vi "Software Echarpe.vi"() -> ()   [LabVIEW 2012]
doc: "Este é o VI principal que contém a interface de controle do espectrógrafo e demais intrumentos."
uses:
  Application/Application.lvclass
  Application/Application.lvclass/Application.ctl
  RxTx/RxTx.lvclass/RxTx.ctl
  Setup File/Setup File.lvclass/Setup File.ctl
  Display Image/Display Image.lvclass/Display Image.ctl
  CCDCamera/CCDCamera.lvclass/CCDCamera.ctl
  Instrument/Instrument.lvclass/Instrument.ctl
  Setup File/Setup File.lvclass
  Display Image/Display Image.lvclass
  CCDCamera/CCDCamera.lvclass
  RxTXCamera/RxTxCamera.lvclass
  State Machine/State Machine.lvclass
  User/User.lvclass
  TCS/TCS.lvclass
  Guider/Guider.lvclass
  Calibration Unit/Calibration Unit.lvclass
  Weather Station/Weather Station.lvclass
  Fore Optics/Fore Optics.lvclass
  Dome/Dome.lvclass
  Instrument/Instrument.lvclass
  RxTx/RxTx.lvclass
panel:
  in  "Image Format":string
  in  "Clean Error":bool
  in  "Application.lvclass":refnum<class "Application.lvclass">
  in  "Night Directory":string="C:\\Users\\Sparc4_2\\Desktop\\Software Echarpe\\Imagens"
  in  "Program ID":string="UNDEFINED"
  in  "Object":string="UNDEFINED"
  in  "Observer":string="ECHARPE"
  in  "Texp Azul":dbl
  in  "Texp Vermelho":dbl
  in  "Posição do rotor":dbl
  in  "Ângulo de paralaxe":dbl
  in  "Blank Button 7":bool
  in  "Blank Button 6":bool
  out "Guiando":bool=TRUE
  out "Waveform Graph":dbl[](graph)
  out "Intensity Graph 4":dbl[][](graph)
  out "Date":string="04/05/2018"
  out "UT":string="2017-10-01T20:34:3 6.000"
  out "Sidereal Time":string="2017-10-01T20:34:3 6.000"
  out "Focus":string="-3.53"
  out "PA":string="14.6415392418"
  out "HA":string="+01:13:05.98"
  out "DEC":string="+00:00:00.000"
  out "Air Mass":string="1.085"
  out "RA":string="00:00:00.000"
  in  "Stop Button":bool
  in  "Interface de controle":T1(tab)
  in  "Pausar":bool
  out "Temperature":i16
  out "Initialization":bool
  out "% Acquired":dbl
  out "Exposing":bool=TRUE
  out "Exposições realizadas":u8(slide) scale=0.0..100.0
  in  "Image Name":string
  in  "# Exposure":dbl
  in  "Exposure time":dbl
  out "% Acquired":dbl
  out "LED sky":bool
  in  "Sky Fiber":bool
  out "LED cal":bool
  in  "Calibration Fiber":bool
  out "Setup File Path:":string
  in  "Read mode":enum32{"No Selection", "1", "2", "3"}(radio)=enum."1"
  in  "Load Setup":bool
  in  "COMP":bool
  in  "FLAT":bool
  in  "Sync Mode":bool
  in  "Adquirir 4":bool
  out "Exposing":bool
  out "Exposições realizadas":u8(slide) scale=0.0..1.0
  in  "Data:":dbl
  in  "Y :":dbl
  in  "X :":dbl
  out "Data:":u32
  out "Y :":u16
  in  "Pausar 3":bool
  in  "Stop 3":bool
  in  "Abort 3":bool
  in  "Adquirir 3":bool
  in  "Pausar 2":bool
  in  "Stop 2":bool
  in  "Stop":bool
  in  "Abort 2":bool
  in  "Adquirir":bool
  in  "Abort":bool
  out "Last Image":string
  in  "# Exposure":u32=1 min=1
  in  "Exposure time":dbl min=0.0
  out "Intensity Graph 2":dbl[][](graph)
  in  "BIAS":bool
  out "X :":u16
  out "Error led":bool
  out "Error Num":u16
  out "Error string":string
  out "Error led 2":bool
  out "Error string 2":string
  out "Error Num 2":u16
  out "Image Graph":i32[][](graph)
  in  "Load Seup 2":bool
  in  "Save Setup":bool
  in  "Tab Control":T2(tab)
  in  "RED Channel Setup":enum32{"Setup", "Binning", "Saving "}(tab)
  in  "Exposure Time (s)  2":dbl
  in  "Acquisition Mode":u16(ring)=1 items=["RESERVED", "Single Scan", "Accumulate", "Kinetics", "Fast Kinetics", "Run Til Abort", "RESERVED", "RESERVED", "RESERVED", "RESERVED", "Time Delayed Integration"]
  in  "Read Mode":u16(ring)=4 items=["Full Vertical Binning", "Multi-Track", "Random-Track", "Single-Track", "Image"]
  in  "Trigger":u16(ring) items=["Internal", "External", "N/A", "N/A", "N/A", "N/A", "External Start", "External Exposure (bulb)", "N/A", "External FVB EM", "Software", "N/A", "External Charge Shifting"]
  in  "Readout Rate":u8(ring) items=["100 KHz at 16 bit", "1 MHz at 16 bit"]
  in  "Vertical Shift Speed":u8(ring) items=["0.6", "2.2", "3.6", "4.33"]
  in  "Vertical clock\nvoltage amplitude":u8
  in  "Pre-amplifier gain":u8(ring)=1 items=["1", "2", "4"]
  in  "Time to close (ms)":u16=50 min=50
  in  "Time to open (ms)":u16=50 min=50
  in  "Shutter TTL":u16(ring) items=["TTL Low", "TTL High"]
  in  "Shutter Mode":u16(ring)=2 items=["Fully Auto", "OPEN", "CLOSED"]
  out "Temperature ºC":dbl(slide) min=-120.0 max=20.0
  in  "Set temperature":i8=20 min=0 max=0
  in  "Cooler ON/OFF":u16(ring) items=["Cooler OFF", "Cooler ON"]
  in  "Vertical binning":u16=1 min=1
  in  "Horizontal binning":u16=1 min=1
  in  "Final Column":u16=1024 min=1
  in  "Final Line":u16=1024 min=1
  in  "Initial Column":u16=1 min=1
  in  "Initial Line":u16=1 min=1
  in  "Sub Image":T3(radio)=enum."1024 x 1024"
  out "Binning":cluster{dbl, dbl}[](graph)
  in  "FITS Format":u16(ring) items=["Unsigned 16", "Unsigned 32", "Signed 16", "Signed 32", "Float"]
  in  "FITS":bool
  in  "SIF":bool
  in  "TIFF":bool
  in  "Tiff Type":u16(ring) items=["8-bit", "16-bit", "Color"]
  in  "Tiff Position":u16=1
  in  "Exposure Time (s)":sgl format="%.2f"
  in  "Acquisition Mode":u16(ring)=1 items=["RESERVED", "Single Scan", "Accumulate", "Kinetics", "Fast Kinetics", "Run Til Abort", "RESERVED", "RESERVED", "RESERVED", "RESERVED", "Time Delayed Integration"]
  in  "Read Mode":u16(ring)=4 items=["Full Vertical Binning", "Multi-Track", "Random-Track", "Single-Track", "Image"]
  in  "Conventional/EM":i32(ring) items=["Conventional", "EM Gain"]
  in  "Trigger":u16(ring) items=["Internal", "External", "N/A", "N/A", "N/A", "N/A", "External Start", "External Exposure (bulb)", "N/A", "External FVB EM", "Software", "N/A", "External Charge Shifting"]
  in  "Readout Rate":i32
  in  "Vertical Shift Speed":i32
  in  "Vertical clock\n  voltage amplitude":i32
  in  "Pre-amplifier gain":i32=1
  in  "EM Gain":bool
  in  "EM Gain  level":i32=1
  in  "EM Advanced 3":bool
  in  "Baseline Clamp 3":bool
  in  "Time to close (ms)":dbl=50.0
  in  "Time to open (ms)":dbl=50.0
  in  "Shutter TTL":u16(ring) items=["TTL Low", "TTL High"]
  in  "Shutter Mode":u16(ring)=2 items=["Fully Auto", "OPEN", "CLOSED"]
  out "Temperature ºC":dbl(slide) scale=-100.0..30.0
  in  "Set temperature":dbl=20.0 min=-80.0 max=20.0
  in  "Cooler ON/OFF":u16(ring) items=["Cooler OFF", "Cooler ON"]
  # "Error Message"
  # "Error Message"
  # "Sync Mode"
  # "Bias"
  # "Flat"
  # "Comp"
  # "RED Channel"
  # "Set Shutter Configuration"
  # "Timings"
  # "Vertical pixel shift"
  # "(TTL level required \nto open  your \nexternal shutter)"
  # "Time to open/close shutter"
  # "Horizontal pixel shift"
  # "Temperature"
  # "Save As:"
  # "BLUE Channel"
  # "Set Shutter Configuration"
  # "Timings"
  # "Vertical pixel shift"
  # "(TTL level required to open \nyour external shutter)"
  # "Time to open/close shutter"
  # "Horizontal pixel shift"
  # "Temperature"
  # "Electron Multiplier (EM) Gain"
  # "Baseline"
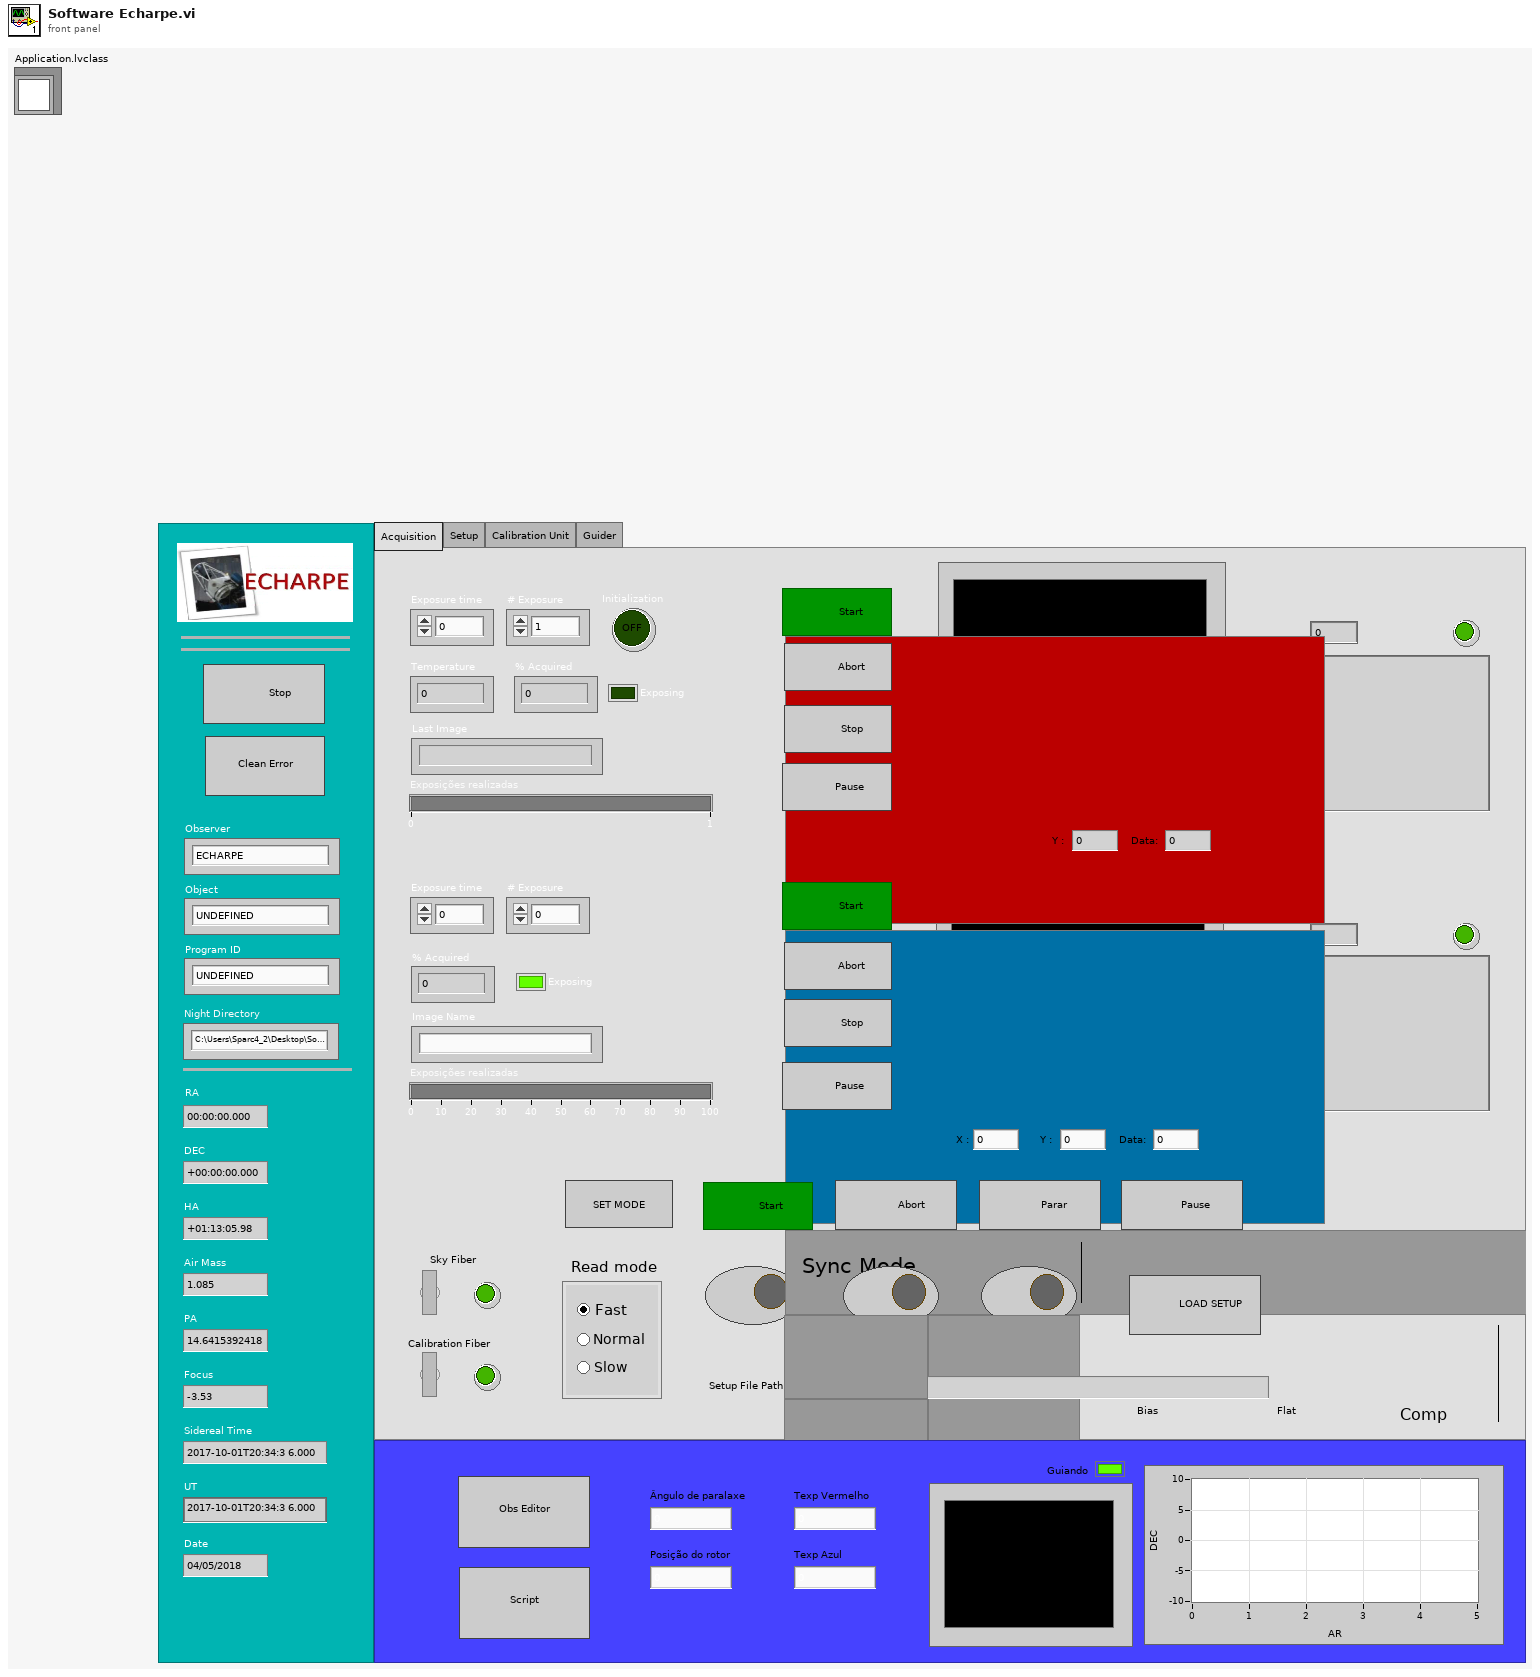
[diagram p1: front panel]
types:
  T1 = enum32{"Acquisition", "Setup", "Calibration Unit", "Guider"}
  T2 = enum32{"RED Channel", "BLUE Channel", "Instrument"}
  T3 = enum32{"256 x 256", "512 x 512", "1024 x 1024", "Custom", "128 x 128", "64 x 64"}
  T4 = cluster{"Currently Temperature":dbl, "Last Image":string, "% Acquired":dbl, "Initilizarion":bool, "Exposing":bool, "Temperature Status":string, "X length":dbl, "Y length":dbl, "Min Temperature":dbl, "Max Temperature":dbl}
  T5 = cluster{"BIAS":refnum<vi>, "FLAT":refnum<vi>, "COMP":refnum<vi>, "Read mode":refnum<vi>}
  T6 = cluster{"Shutter Mode ":u16, "Pre-amplifier gain":i32, "Vertical Shift Speed":i32, "Readout Rate ":i32, "Exposure Time (s) ":sgl}
  T7 = cluster{"Cooler ON/OFF":u16, "Set temperature":dbl, "Shutter Mode ":u16, "Shutter TTL":u16, "Time to open (ms)":dbl, "Time to close (ms)":dbl, "Pre-amplifier gain":i32, "Vertical clock\n  voltage amplitude":i32, "Vertical Shift Speed":i32, "Readout Rate ":i32, "Trigger ":u16, "Conventional/EM":i32, "Read Mode ":u16, "Acquisition Mode ":u16, "Exposure Time (s) ":sgl, "Initial Line":i32, "Initial Column":i32, "Final Line":i32, "Final Column":i32, "Horizontal binning":i32, "Vertical binning ":i32, "FITS Format":u16, "Image Format":string, "Tiff Position ":u16, "Tiff Type":u16, "Image Path":string}
  T8 = cluster{"DSTATUS":string, "DPOS":string, "DTEMP":string, "DHUM":string, "DLAMP":string, "DFLAT":string}
  T9 = cluster{"ADC":string, "ADCSPEED":string, "CALMIRR":string}
  T10 = cluster{"TEMPEXT":string, "PRESSURE":string, "HUMIDITY":string, "WINDDIR":string, "WSPEED":string}
  T11 = cluster{"THARLAMP":string, "HALLAMP":string, "AGITATOR":string, "THARMIRR":string}
  T12 = cluster{"GUIDING":string, "GUIDTEXP":string, "GUIDFREQ":string, "GUIDOBJX":string, "GUIDOBJY":string, "AVGYCOOR":string, "AVGXCORR":string, "GFOCUS":string}
  T13 = cluster{"Observation type":string, "Read Mode":string, "Sky fiber":bool, "Calibration fiber":bool, "Sync Mode":string, "Date":string}
  T14 = cluster{"RA":string, "DEC":string, "TELRA":string, "TELDEC":string, "RA_DEG":string, "DEC_DEG":string, "Epoch":string, "AirMass":string, "Initial Air Mass":string, "HA":string, "HAD":string, "Final Air Mass":string, "X Offset":string, "Y Offset":string, "PA":string, "Camera Focus":string, "TCS Focus":string, "Moon distance":string, "Moon height":string, "Moon Phase":string, "TCSST":string, "TCSUT":string}
  T15 = cluster{"Observer":string, "Object":string, "Program ID":string, "Night Directory":string}
  T16 = cluster{"Read Mode":string, "Acquisition Mode":string, "Trigger":string, "Exposure Time":string, "VShift Speed":string, "Readout rate":string, "Pre amp":string, "Shutter Mode":string, "Shutter TTL":string, "Time to open shutter":string, "Time to close shutter":string, "Cooler":string, "Temperature":string, "Initial Line":string, "Initial Column":string, "Final Line":string, "Final Column":string, "Horizontal binning":string, "Vertical binning":string, "Sub image":string}
  T17 = enum8{"Enabled", "Disabled", "Disabled and Grayed Out"}
  T18 = cluster{"Exposing":bool, "% Acquired":dbl, "Initialization":bool, "CurrentlyTemp":i16, "Exposições realizadas":u8, "Image Graph":i32[][], "Temperature Status":string, "Last Image":string}
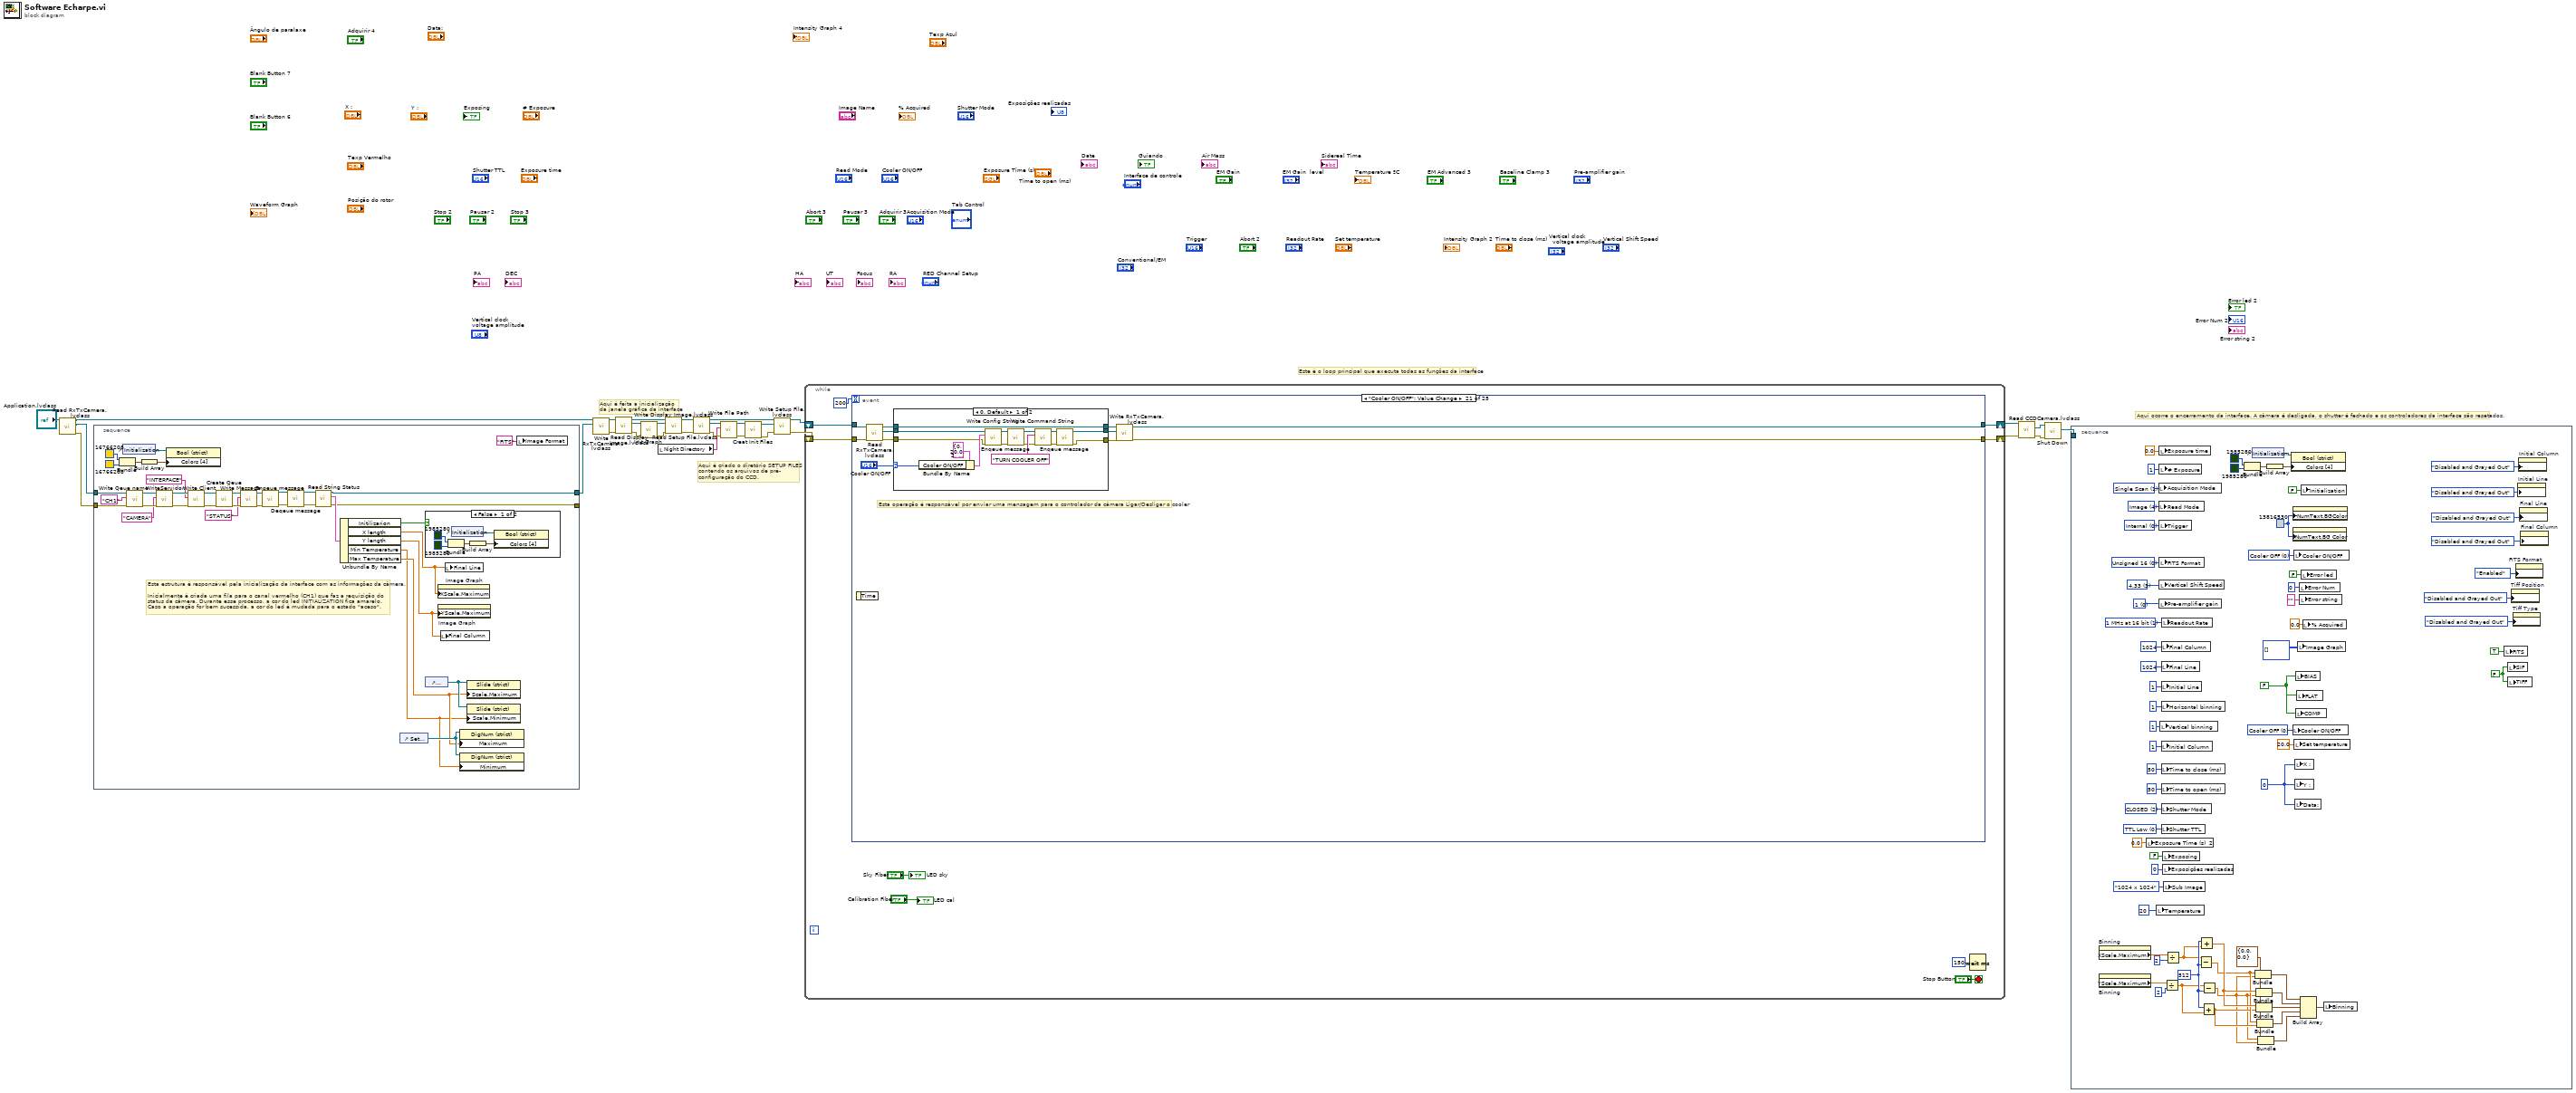
[diagram p0: block diagram]
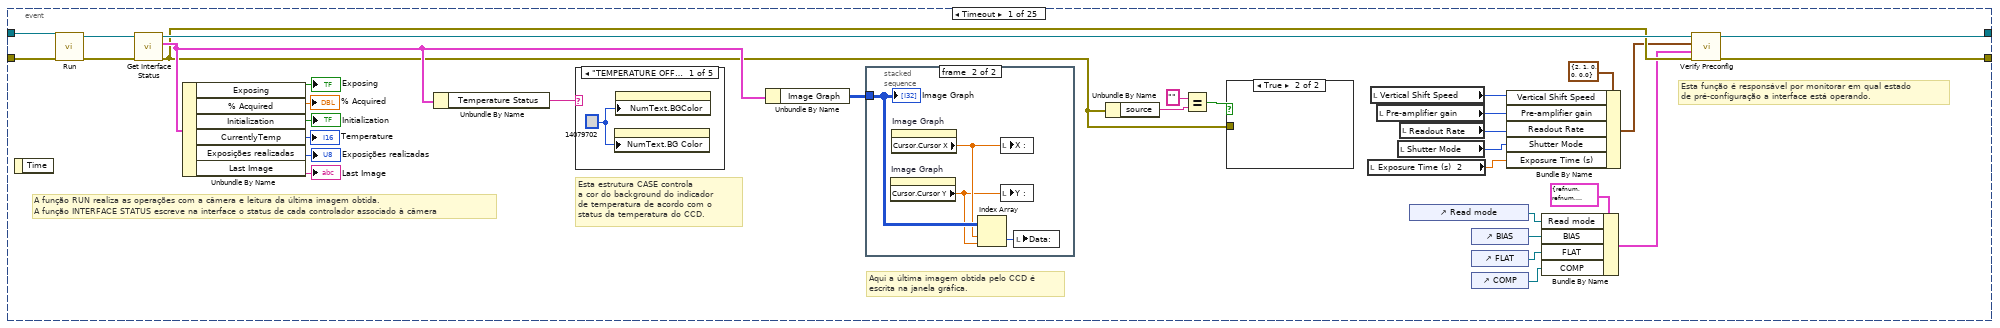
[diagram p2: hidden frame]
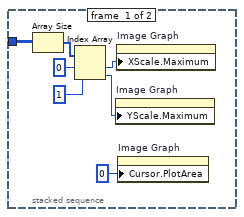
[diagram p3: hidden frame]
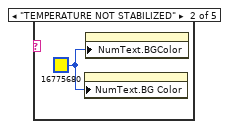
[diagram p4: hidden frame]
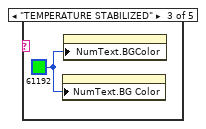
[diagram p5: hidden frame]
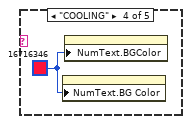
[diagram p6: hidden frame]
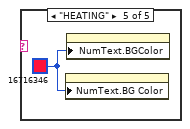
[diagram p7: hidden frame]
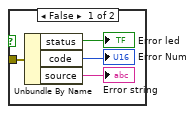
[diagram p8: hidden frame]
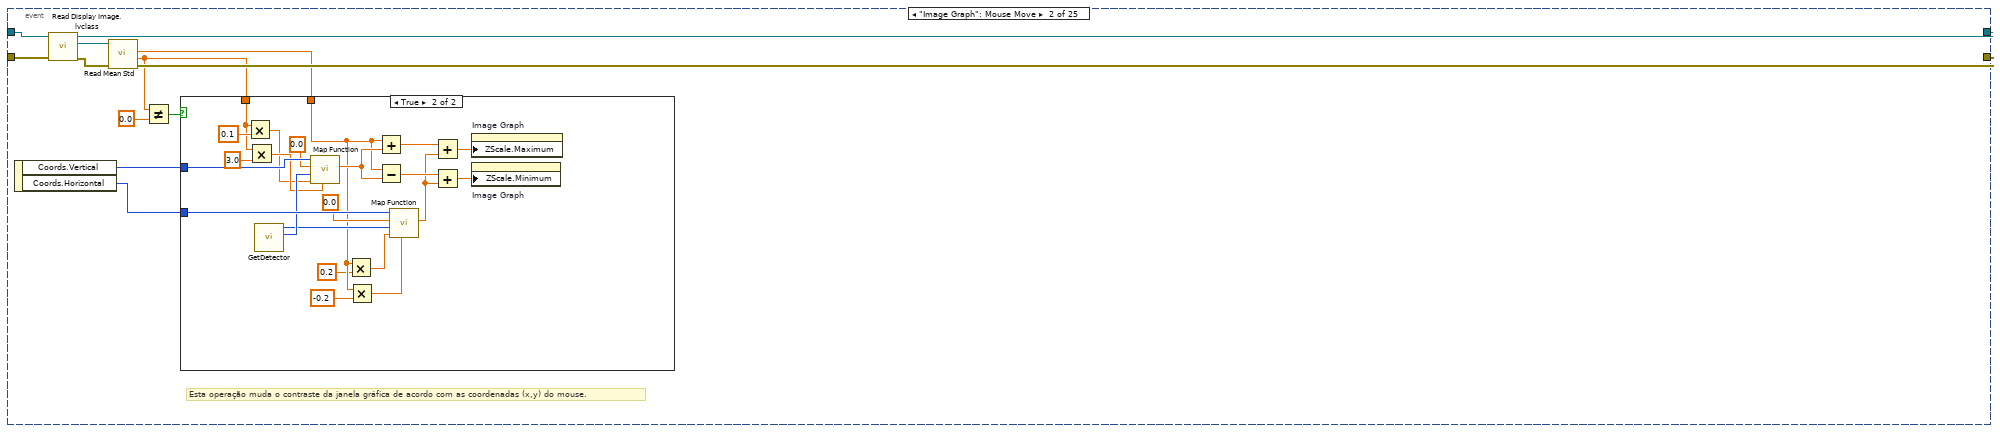
[diagram p9: hidden frame]
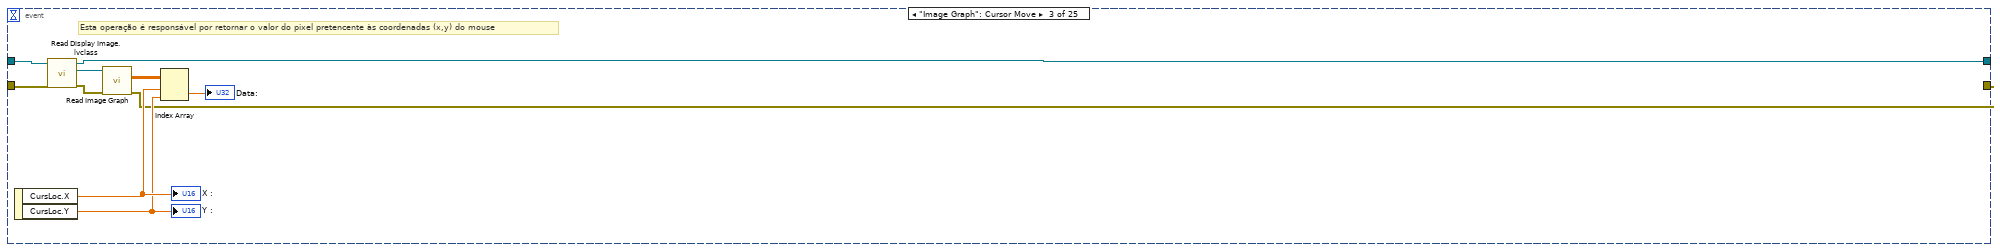
[diagram p11: hidden frame]
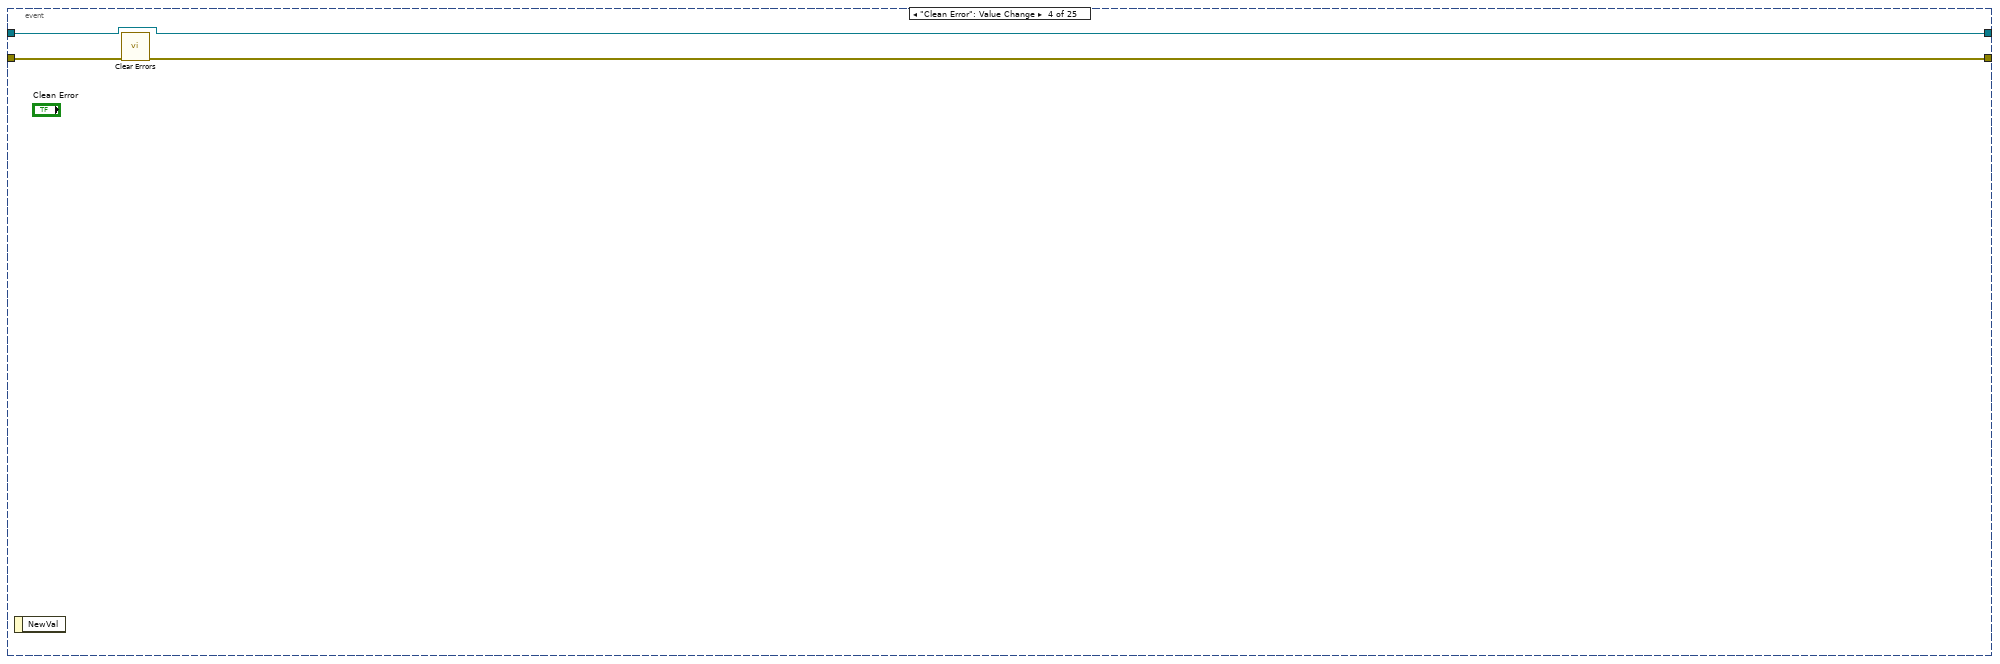
[diagram p12: hidden frame]
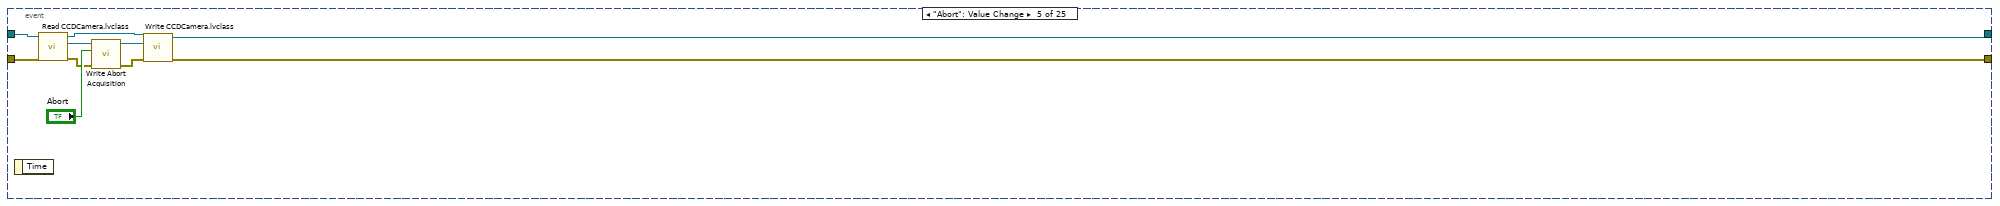
[diagram p13: hidden frame]
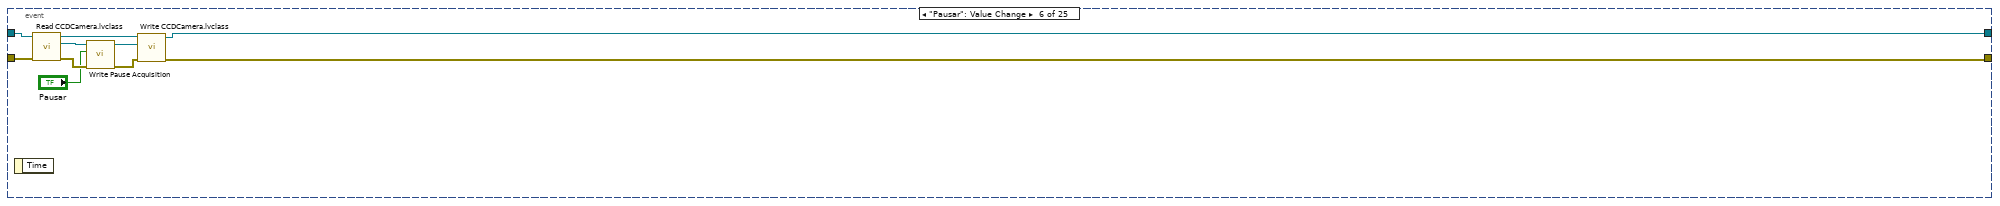
[diagram p14: hidden frame]
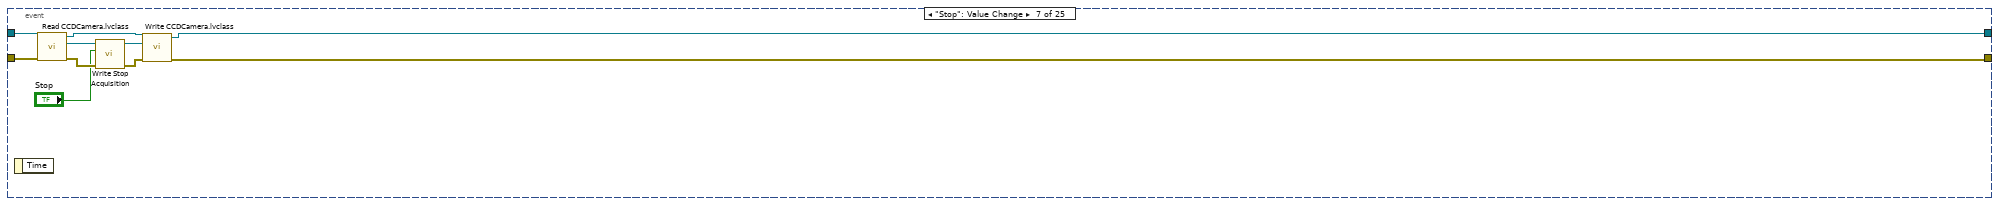
[diagram p15: hidden frame]
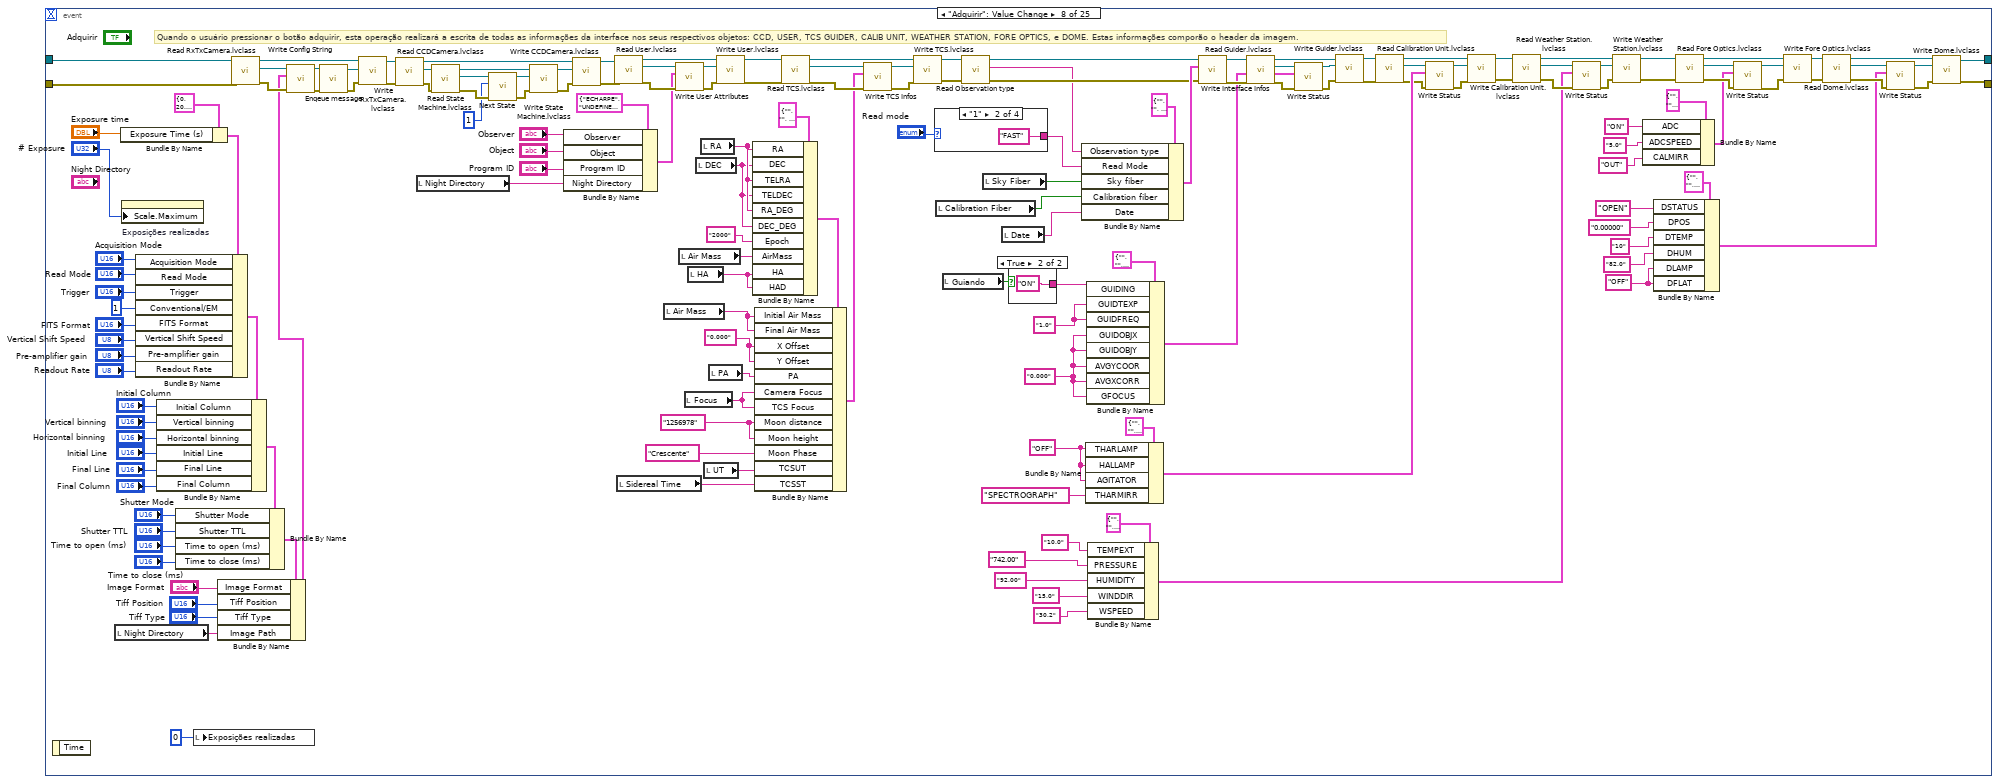
[diagram p16: hidden frame]
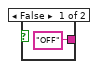
[diagram p17: hidden frame]
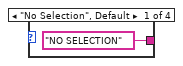
[diagram p18: hidden frame]
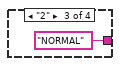
[diagram p19: hidden frame]
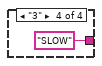
[diagram p20: hidden frame]
diagram:
  # "Aqui ocorre o encerramento da interface. A câmera é desligada, o shutter é fechado e os controladores da interface são resetados."
  # "Este é o loop principal que executa todas as funções da interface"
  # "Aqui é criado o diretório SETUP FILES\ncontendo os arquivos de pré-\nconfiguração do CCD."
  # "Aqui é feita a inicialização \nda janela gráfica da interface"
  n1 = call "Read RxTxCamera.lvclass.vi"("Application in"="Application.lvclass") -> ("error out"=w5:errorcluster, "RxTxCamera.lvclass"=w6:refnum<class "RxTxCamera.lvclass">, "Application out"=w2:refnum<class "Application.lvclass">)  [unwired: 8 in]
  n2 = stacked-sequence {
    tunnel: [w38] -> w1
    tunnel: w5 -> [w51]
    tunnel: w6 -> [w50]
    tunnel: [w39] -> _
    frame #0 {
      # "Esta estrutura é responsável pela inicialização da interface com as informações da câmera.\n\nInicialmente é criada uma fila para o canal vermelho (CH1) que faz a requisição do\nstatus da câmera. Durante esse processo, a cor do led INITIALIZATION fica amarelo.\nCaso a operação for bem sucessida, a cor do led é mudada para o estado \"aceso\"."
      n3 = Bundle(u32 16766208, u32 16766208) -> (w61:cluster{u32, u32})  [unwired: 1 in]
      n4 = control-ref of="Initialization"() -> (w65:refnum<vi>)
      n5 = call "Write Qeue name.vi"("error in (no error)"=w51, "Qeue name"="CH1", "RxTx in"=w50) -> ("error out"=w36:errorcluster, "RxTx out"=w37:refnum<class "RxTxCamera.lvclass">)  [unwired: 7 in]
      n6 = Build Array(w61) -> (w64:cluster{u32, u32}[])
      n7 = call "WriteServidor.vi"("error in (no error)"=w36, "Servidor"="CAMERA" ("Qeue name"), "RxTx in"=w37) -> ("error out"=w35:errorcluster, "RxTx out"=w32:refnum<class "RxTxCamera.lvclass">)  [unwired: 7 in]
      n8 = property on="Property Node" class="Bool (strict)"(reference=w65, "Colors [4]"=w64) -> ()  [unwired: 1 in, 2 out]
      n9 = call "Write Client.vi"("error in (no error)"=w35, "Client"="INTERFACE" ("Qeue name"), "RxTx in"=w32) -> ("error out"=w34:errorcluster, "RxTx out"=w33:refnum<class "RxTxCamera.lvclass">)  [unwired: 7 in]
      n10 = call "Create Qeue.vi"("error in (no error)"=w34, "RxTx in"=w33) -> ("error out"=w57:errorcluster, "RxTx out"=w56:refnum<class "RxTxCamera.lvclass">)  [unwired: 8 in]
      n11 = call "Write Message.vi"("error in (no error)"=w57, "Message"="STATUS" ("Qeue name"), "RxTx in"=w56) -> ("error out"=w54:errorcluster, "RxTx out"=w55:refnum<class "RxTxCamera.lvclass">)  [unwired: 7 in]
      n12 = call "Enqeue message.vi"("error in (no error)"=w54, "RxTx in"=w55) -> ("error out"=w58:errorcluster, "RxTx out"=w59:refnum<class "RxTxCamera.lvclass">)  [unwired: 8 in]
      n13 = call "Deqeue message.vi"("error in (no error)"=w58, "RxTx in"=w59) -> ("error out"=w49:errorcluster, "RxTx out"=w48:refnum<class "RxTxCamera.lvclass">)  [unwired: 8 in]
      n14 = call "Read String Status.vi"("error in (no error)"=w49, "RxTxCamera in"=w48) -> ("error out"=w39:errorcluster, "Camera Status"=w47:T4, "RxTxCamera out"=w38:refnum<class "RxTxCamera.lvclass">)  [unwired: 7 in]
      n15 = Unbundle By Name(w47) -> ("Initilizarion"=w46:bool, "X length"=w45:dbl, "Y length"=w44:dbl, "Min Temperature"=w40:dbl, "Max Temperature"=w41:dbl)
      n16 = control-ref of="Set temperature"() -> (w42:refnum<vi>)
      n17 = control-ref of="Temperature ºC"() -> (w43:refnum<vi>)
      n18 = case shown="False" w46 {
        frame False {
          n19 = Bundle(u32 1985280, u32 1985280) -> (w70:cluster{u32, u32})  [unwired: 1 in]
          n20 = control-ref of="Initialization"() -> (w66:refnum<vi>)
          n21 = Build Array(w70) -> (w67:cluster{u32, u32}[])
          n22 = property on="Property Node" class="Bool (strict)"(reference=w66, "Colors [4]"=w67) -> ()  [unwired: 1 in, 2 out]
        }
        frame True {
          n23 = Bundle(u32 6618880, u32 6618880) -> (w75:cluster{u32, u32})  [unwired: 1 in]
          n24 = control-ref of="Initialization"() -> (w71:refnum<vi>)
          n25 = Build Array(w75) -> (w72:cluster{u32, u32}[])
          n26 = property on="Property Node" class="Bool (strict)"(reference=w71, "Colors [4]"=w72) -> ()  [unwired: 1 in, 2 out]
        }
      }
      n27 = property on="Image Graph" class="IntGraph (strict)"("XScale.Maximum"=w45) -> ()  [unwired: 2 in, 2 out]
      n28 = property on="Image Graph" class="IntGraph (strict)"("YScale.Maximum"=w44) -> ()  [unwired: 2 in, 2 out]
      n29 = local write "Final Column"(w44) -> ()
      n30 = local write "Final Line"(w45) -> ()
      n31 = property class="DigNum (strict)"(reference=w42, "Maximum"=w41) -> ()  [unwired: 1 in, 2 out]
      n32 = property class="DigNum (strict)"(reference=w42, "Minimum"=w40) -> ()  [unwired: 1 in, 2 out]
      n33 = property class="Slide (strict)"(reference=w43, "Scale.Maximum"=w41) -> ()  [unwired: 1 in, 2 out]
      n34 = property class="Slide (strict)"(reference=w43, "Scale.Minimum"=w40) -> ()  [unwired: 1 in, 2 out]
      n35 = local write "Image Format"("FITS" ("Image Format")) -> ()
    }
  }
  n36 = call "Write RxTxCamera.lvclass.vi"("RxTxCamera.lvclass"=w1, "Application in"=w2) -> ("error out"=w3:errorcluster, "Application out"=w4:refnum<class "Application.lvclass">)  [unwired: 8 in]
  n37 = call "Read Display Image.lvclass.vi"("error in (no error)"=w3, "Application in"=w4) -> ("error out"=w24:errorcluster, "Display Image.lvclass"=w23:refnum<class "Display Image.lvclass">, "Application out"=w20:refnum<class "Application.lvclass">)  [unwired: 7 in]
  n38 = call "Init Graph.vi"("error in (no error)"=w24, "Display Image in"=w23) -> ("error out"=w21:errorcluster, "Display Image out"=w22:refnum<class "Display Image.lvclass">)  [unwired: 8 in]
  n39 = local read "Night Directory"() -> (w15:string)
  n40 = call "Write Display Image.lvclass.vi"("error in (no error)"=w21, "Display Image.lvclass"=w22, "Application in"=w20) -> ("error out"=w19:errorcluster, "Application out"=w18:refnum<class "Application.lvclass">)  [unwired: 7 in]
  n41 = call "Read Setup File.lvclass.vi"("error in (no error)"=w19, "Application in"=w18) -> ("error out"=w17:errorcluster, "Setup File.lvclass"=w16:refnum<class "Setup File.lvclass">, "Application out"=w10:refnum<class "Application.lvclass">)  [unwired: 7 in]
  n42 = call "Write File Path.vi"("error in (no error)"=w17, "File Path"=w15, "Setup File in"=w16) -> ("error out"=w14:errorcluster, "Setup File out"=w13:refnum<class "Setup File.lvclass">)  [unwired: 7 in]
  n43 = call "Creat Init Files.vi"("error in (no error)"=w14, "Setup File in"=w13) -> ("error out"=w12:errorcluster, "Setup File out"=w11:refnum<class "Setup File.lvclass">)  [unwired: 8 in]
  n44 = call "Write Setup File.lvclass.vi"("error in (no error)"=w12, "Setup File.lvclass"=w11, "Application in"=w10) -> ("error out"=w9:errorcluster, "Application out"=w8:refnum<class "Application.lvclass">)  [unwired: 7 in]
  n45 = while {
    shift-right: [w81] -> w27
    shift-left: w8 -> [w82]
    shift-right: [w80] -> w28
    shift-left: w9 -> [w83]
    stop <- "Stop Button" stop-if-true
    n46 = event shown="[20] \"Cooler ON/OFF\": Value Change" {
      selector: _ -> [_ _ _ _ _ _ _ _ _ _ _ _ _ _ _ _ _ _ _ _ _ _ _ _ _]
      dyn-events: _ -> [_ _ _ _ _ _ _ _ _ _ _ _ _ _ _ _ _ _ _ _ _ _ _ _ _]
      timeout: 200 -> [_ _ _ _ _ _ _ _ _ _ _ _ _ _ _ _ _ _ _ _ _ _ _ _ _]
      tunnel: w83 -> [w117 w149 w181 w184 w194 w197 w209 w228 w403 w445 w751 w803 w922 w931 w940 w949 w964 w983 w985 w988 w997 w1035 w1131 w1139 _]
      tunnel: w82 -> [w85 w148 w180 w183 w193 w198 w208 w227 w402 w444 w750 w802 w921 w930 w939 w948 w963 w982 w984 w987 w996 w1034 w1130 w1138 w1152]
      tunnel: [w102 w145 w173 w183 w185 w195 w205 w262 w393 w438 w705 w802 w921 w930 w939 w948 w961 w966 w984 w987 w991 w1036 w1126 w1135 w1143] -> w81
      tunnel: [w100 w144 w172 w182 w186 w196 w206 w263 w394 w436 w706 w803 w922 w931 w940 w949 w962 w967 w985 w988 w990 w1037 w1127 w1136 w1142] -> w80
      event Timeout {
        # "Esta função é responsável por monitorar em qual estado\nde pré-configuração a interface está operando."
        # "Aqui a última imagem obtida pelo CCD é \nescrita na janela gráfica."
        # "Esta estrutura CASE controla\na cor do background do indicador\nde temperatura de acordo com o \nstatus da temperatura do CCD."
        # "A função RUN realiza as operações com a câmera e leitura da última imagem obtida.\nA função INTERFACE STATUS escreve na interface o status de cada controlador associado à câmera"
        n47 = event-data() -> ()  [unwired: 1 in, 1 out]
        n48 = call "Run.vi"("error in (no error)"=w117, "Application in"=w85) -> ("error out"=w116:errorcluster, "Application out"=w115:refnum<class "Application.lvclass">)  [unwired: 8 in]
        n49 = call "Get Interface Status.vi"("error in (no error)"=w116, "Application in"=w115) -> ("error out"=w101:errorcluster, "RED panel Cluster"=w105:T18, "Application out"=w103:refnum<class "Application.lvclass">)  [unwired: 7 in]
        n50 = Unbundle By Name(w105) -> ("Exposing"=→"Exposing":bool, "% Acquired"=→"% Acquired":dbl, "Initialization"=→"Initialization":bool, "CurrentlyTemp"=→"Temperature":i16, "Exposições realizadas"=→"Exposições realizadas":u8, "Last Image"=→"Last Image":string)
        n51 = Unbundle By Name(w105) -> ("Temperature Status"=w106:string)
        n52 = case shown="\"TEMPERATURE OFF\", Default" w106 {
          frame "TEMPERATURE OFF", Default {
            w129 = u32 14079702
            n53 = property on="Temperature" class="DigNum (strict)"("NumText.BG Color"=w129) -> ()  [unwired: 2 in, 2 out]
            n54 = property on="Temperature" class="DigNum (strict)"("NumText.BGColor"=w129) -> ()  [unwired: 2 in, 2 out]
          }
          frame "TEMPERATURE NOT STABILIZED" {
            w130 = u32 16775680
            n55 = property on="Temperature" class="DigNum (strict)"("NumText.BG Color"=w130) -> ()  [unwired: 2 in, 2 out]
            n56 = property on="Temperature" class="DigNum (strict)"("NumText.BGColor"=w130) -> ()  [unwired: 2 in, 2 out]
          }
          frame "TEMPERATURE STABILIZED" {
            w131 = u32 61192
            n57 = property on="Temperature" class="DigNum (strict)"("NumText.BG Color"=w131) -> ()  [unwired: 2 in, 2 out]
            n58 = property on="Temperature" class="DigNum (strict)"("NumText.BGColor"=w131) -> ()  [unwired: 2 in, 2 out]
          }
          frame "COOLING" {
            w132 = u32 16716346
            n59 = property on="Temperature" class="DigNum (strict)"("NumText.BG Color"=w132) -> ()  [unwired: 2 in, 2 out]
            n60 = property on="Temperature" class="DigNum (strict)"("NumText.BGColor"=w132) -> ()  [unwired: 2 in, 2 out]
          }
          frame "HEATING" {
            w133 = u32 16716346
            n61 = property on="Temperature" class="DigNum (strict)"("NumText.BG Color"=w133) -> ()  [unwired: 2 in, 2 out]
            n62 = property on="Temperature" class="DigNum (strict)"("NumText.BGColor"=w133) -> ()  [unwired: 2 in, 2 out]
          }
        }
        n63 = Unbundle By Name(w105) -> ("Image Graph"=w104:i32[][])
        n64 = stacked-sequence {
          tunnel: w104 -> [w124 w128]
          frame #0 {
            n65 = Array Size(array=w124) -> (size(s)=w123:i32[])
            n66 = Index Array(array=w123, index #1=0 ("index"), index #2=1 ("index")) -> (element #1=w122:i32, element #2=w121:i32)
            n67 = property on="Image Graph" class="IntGraph (strict)"("YScale.Maximum"=w121) -> ()  [unwired: 2 in, 2 out]
            n68 = property on="Image Graph" class="IntGraph (strict)"("XScale.Maximum"=w122) -> ()  [unwired: 2 in, 2 out]
            n69 = property on="Image Graph" class="IntGraph (strict)"("Cursor.PlotArea"=0 ("Cursor.Plot Area")) -> ()  [unwired: 2 in, 2 out]
          }
          frame #1 {
            n70 = property on="Image Graph" class="IntGraph (strict)"() -> ("Cursor.Cursor Y"=w126:dbl)  [unwired: 2 in, 2 out]
            n71 = property on="Image Graph" class="IntGraph (strict)"() -> ("Cursor.Cursor X"=w127:dbl)  [unwired: 2 in, 2 out]
            n72 = Index Array(array=w128, index (row)=w127, index (col)=w126) -> (element=w125:i32)
            n73 = local write "X :"(w127) -> ()
            n74 = local write "Y :"(w126) -> ()
            n75 = local write "Data:"(w125) -> ()
            "Image Graph" <- w128
          }
        }
        n76 = Unbundle By Name(w101) -> ("source"=w114:string)
        n77 = Equal?(x="", y=w114) -> (x = y?=w112:bool)
        n78 = case shown="True" w112 {
          tunnel: w101 -> [w134 _]
          frame False {
            n79 = Unbundle By Name(w134) -> ("status"=→"Error led":bool, "code"=→"Error Num":i32, "source"=→"Error string":string)
          }
          frame True {
          }
        }
        n80 = local read "Exposure Time (s)  2"() -> (w97:dbl)
        n81 = local read "Vertical Shift Speed"() -> (w93:u8)
        n82 = local read "Pre-amplifier gain"() -> (w94:u8)
        n83 = local read "Shutter Mode"() -> (w96:u16)
        n84 = local read "Readout Rate"() -> (w95:u8)
        n85 = control-ref of="Read mode"() -> (w92:refnum<vi>)
        n86 = control-ref of="BIAS"() -> (w89:refnum<vi>)
        n87 = control-ref of="FLAT"() -> (w88:refnum<vi>)
        n88 = control-ref of="COMP"() -> (w87:refnum<vi>)
        n89 = Bundle By Name(cluster=T6 {"Shutter Mode "=2, "Pre-amplifier gain"=1, "Vertical Shift Speed"=0, "Readout Rate "=0, "Exposure Time (s) "=0.0} ("RED Channel Settings"), "Vertical Shift Speed"=w93, "Pre-amplifier gain"=w94, "Readout Rate"=w95, "Shutter Mode"=w96, "Exposure Time (s)"=w97) -> (w99:T6)
        n90 = Bundle By Name(cluster=T5 {"BIAS"=refnum, "FLAT"=refnum, "COMP"=refnum, "Read mode"=refnum} ("Ref controls"), "Read mode"=w92, "BIAS"=w89, "FLAT"=w88, "COMP"=w87) -> (w91:T5)
        n91 = call "Verify Preconfig.vi"("error in (no error)"=w101, "Ref controls"=w91, "RED Channel Settings"=w99, "Application in"=w103) -> ("error out"=w100:errorcluster, "Application out"=w102:refnum<class "Application.lvclass">)  [unwired: 6 in]
      }
      event "Image Graph": Mouse Move {
        # "Esta operação muda o contraste da janela gráfica de acordo com as coordenadas (x,y) do mouse."
        n92 = event-data() -> ("Coords.Vertical"=w143:i32, "Coords.Horizontal"=w142:i32)  [unwired: 1 in]
        n93 = call "Read Display Image.lvclass.vi"("error in (no error)"=w149, "Application in"=w148) -> ("error out"=w146:errorcluster, "Display Image.lvclass"=w147:refnum<class "Display Image.lvclass">, "Application out"=w145:refnum<class "Application.lvclass">)  [unwired: 7 in]
        n94 = call "Read Mean Std.vi"("error in (no error)"=w146, "Display Image in"=w147) -> ("error out"=w144:errorcluster, "Stddev"=w138:dbl, "Mean"=w141:dbl)  [unwired: 6 in, 1 out]
        n95 = Not Equal?(x=w138, y=0.0) -> (x != y?=w140:bool)
        n96 = case shown="True" w140 {
          tunnel: w138 -> [_ w165]
          tunnel: w143 -> [_ w163]
          tunnel: w142 -> [_ w162]
          tunnel: w141 -> [_ w155]
          frame False {
          }
          frame True {
            n97 = Multiply(x=w165, y=0.1) -> (x*y=w158:dbl)
            n98 = Multiply(x=w165, y=3.0) -> (x*y=w159:dbl)
            n99 = call <userlib>:"GetDetector.vi"() -> ("ypixels"=w161:i32, "xpixels"=w156:i32)  [unwired: 4 in, 2 out]
            n100 = call "Map Function.vi"("Ysup"=w159, "Yinf"=w158, "Xsup"=w161, "Xinf"=0.0 ("Yinf"), "X"=w163) -> ("Value"=w169:dbl)  [unwired: 6 in]
            n101 = Multiply(x=w155, y=0.2) -> (x*y=w153:dbl)
            n102 = Multiply(x=w155, y=-0.2) -> (x*y=w152:dbl)
            n103 = Add(x=w155, y=w169) -> (x+y=w170:dbl)
            n104 = Subtract(x=w155, y=w169) -> (x-y=w171:dbl)
            n105 = call "Map Function.vi"("Ysup"=w152, "Yinf"=w153, "Xsup"=w156, "Xinf"=0.0 ("Yinf"), "X"=w162) -> ("Value"=w150:dbl)  [unwired: 6 in]
            n106 = Add(x=w170, y=w150) -> (x+y=w167:dbl)
            n107 = Add(x=w171, y=w150) -> (x+y=w166:dbl)
            n108 = property on="Image Graph" class="IntGraph (strict)"("ZScale.Maximum"=w167) -> ()  [unwired: 2 in, 2 out]
            n109 = property on="Image Graph" class="IntGraph (strict)"("ZScale.Minimum"=w166) -> ()  [unwired: 2 in, 2 out]
          }
        }
      }
      event "Image Graph": Cursor Move {
        # "Esta operação é responsável por retornar o valor do pixel pretencente às coordenadas (x,y) do mouse"
        n110 = event-data() -> ("CursLoc.X"=w175:dbl, "CursLoc.Y"=w174:dbl)  [unwired: 1 in]
        "Y :" <- w174
        "X :" <- w175
        n111 = call "Read Display Image.lvclass.vi"("error in (no error)"=w181, "Application in"=w180) -> ("error out"=w178:errorcluster, "Display Image.lvclass"=w179:refnum<class "Display Image.lvclass">, "Application out"=w173:refnum<class "Application.lvclass">)  [unwired: 7 in]
        n112 = call "Read Image Graph.vi"("error in (no error)"=w178, "Display Image in"=w179) -> ("error out"=w172:errorcluster, "Image Graph"=w177:dbl[][])  [unwired: 7 in, 1 out]
        n113 = Index Array(array=w177, index (row)=w175, index (col)=w174) -> (element=→"Data:":dbl)
      }
      event "Clean Error": Value Change {
        n114 = event-data() -> ()  [unwired: 1 in, 1 out]
        n115 = call <vilib>:"Clear Errors.vi"("error in (no error)"=w184) -> ("error out"=w182:errorcluster)  [unwired: 6 in]
      }
      event "Abort": Value Change {
        n116 = event-data() -> ()  [unwired: 1 in, 1 out]
        n117 = call "Read CCDCamera.lvclass.vi"("error in (no error)"=w194, "Application in"=w193) -> ("error out"=w191:errorcluster, "CCDCamera.lvclass"=w190:refnum<class "CCDCamera.lvclass">, "Application out"=w187:refnum<class "Application.lvclass">)  [unwired: 7 in]
        n118 = call "Write Abort Acquisition.vi"("error in (no error)"=w191, "Abort Acquisition"="Abort", "CCDCamera in"=w190) -> ("error out"=w189:errorcluster, "CCDCamera out"=w188:refnum<class "CCDCamera.lvclass">)  [unwired: 7 in]
        n119 = call "Write CCDCamera.lvclass.vi"("error in (no error)"=w189, "CCDCamera.lvclass"=w188, "Application in"=w187) -> ("error out"=w186:errorcluster, "Application out"=w185:refnum<class "Application.lvclass">)  [unwired: 7 in]
      }
      event "Pausar": Value Change {
        n120 = event-data() -> ()  [unwired: 1 in, 1 out]
        n121 = call "Read CCDCamera.lvclass.vi"("error in (no error)"=w197, "Application in"=w198) -> ("error out"=w200:errorcluster, "CCDCamera.lvclass"=w203:refnum<class "CCDCamera.lvclass">, "Application out"=w204:refnum<class "Application.lvclass">)  [unwired: 7 in]
        n122 = call "Write Pause Acquisition.vi"("error in (no error)"=w200, "Pause Acquisition"="Pausar", "CCDCamera in"=w203) -> ("error out"=w201:errorcluster, "CCDCamera out"=w202:refnum<class "CCDCamera.lvclass">)  [unwired: 7 in]
        n123 = call "Write CCDCamera.lvclass.vi"("error in (no error)"=w201, "CCDCamera.lvclass"=w202, "Application in"=w204) -> ("error out"=w196:errorcluster, "Application out"=w195:refnum<class "Application.lvclass">)  [unwired: 7 in]
      }
      event "Stop": Value Change {
        n124 = event-data() -> ()  [unwired: 1 in, 1 out]
        n125 = call "Read CCDCamera.lvclass.vi"("error in (no error)"=w209, "Application in"=w208) -> ("error out"=w213:errorcluster, "CCDCamera.lvclass"=w212:refnum<class "CCDCamera.lvclass">, "Application out"=w210:refnum<class "Application.lvclass">)  [unwired: 7 in]
        n126 = call "Write Stop Acquisition.vi"("error in (no error)"=w213, "Stop Acquisition"="Stop", "CCDCamera in"=w212) -> ("error out"=w214:errorcluster, "CCDCamera out"=w211:refnum<class "CCDCamera.lvclass">)  [unwired: 7 in]
        n127 = call "Write CCDCamera.lvclass.vi"("error in (no error)"=w214, "CCDCamera.lvclass"=w211, "Application in"=w210) -> ("error out"=w206:errorcluster, "Application out"=w205:refnum<class "Application.lvclass">)  [unwired: 7 in]
      }
      event "Adquirir": Value Change {
        w235 = "1256978" ("AirMass")
        w236 = "0.000" ("AirMass")
        w252 = "OFF"
        w296 = "OFF"
        w306 = "0.000"
        w307 = "1.0"
        # "Quando o usuário pressionar o botão adquirir, esta operação realizará a escrita de todas as informações da interface nos seus respectivos objetos: CCD, USER, TCS GUIDER, CALIB UNIT, WEATHER STATION, FORE OPTICS, e DOME. Estas informações comporão o header da imagem."
        n128 = event-data() -> ()  [unwired: 1 in, 1 out]
        n129 = local read "Night Directory"() -> (w215:string)
        n130 = Bundle By Name(cluster=T7 {"Cooler ON/OFF"=0, "Set temperature"=20.0, "Shutter Mode "=2, "Shutter TTL"=0, "Time to open (ms)"=50.0, "Time to close (ms)"=50.0, "Pre-amplifier gain"=0, "Vertical clock\n  voltage amplitude"=0, "Vertical Shift Speed"=3, "Readout Rate "=1, "Trigger "=0, "Conventional/EM"=1, "Read Mode "=4, "Acquisition Mode "=1, "Exposure Time (s) "=0.0, "Initial Line"=1, "Initial Column"=1, "Final Line"=1024, "Final Column"=1024, "Horizontal binning"=1, "Vertical binning "=1, "FITS Format"=0, "Image Format"="FITS", "Tiff Position "=1, "Tiff Type"=0, "Image Path"=""} ("RED Channel Settings"), "Exposure Time (s)"="Exposure time") -> (w355:T7)
        n131 = property on="Exposições realizadas" class="Slide (strict)"("Scale.Maximum"="# Exposure") -> ()  [unwired: 2 in, 2 out]
        n132 = Bundle By Name(cluster=w355, "Acquisition Mode"="Acquisition Mode", "Read Mode"="Read Mode", "Trigger"="Trigger", "Conventional/EM"=1, "FITS Format"="FITS Format", "Vertical Shift Speed"="Vertical Shift Speed", "Pre-amplifier gain"="Pre-amplifier gain", "Readout Rate"="Readout Rate") -> (w360:T7)
        n133 = Bundle By Name(cluster=w360, "Initial Column"="Initial Column", "Vertical binning"="Vertical binning", "Horizontal binning"="Horizontal binning", "Initial Line"="Initial Line", "Final Line"="Final Line", "Final Column"="Final Column") -> (w370:T7)
        n134 = Bundle By Name(cluster=w370, "Shutter Mode"="Shutter Mode", "Shutter TTL"="Shutter TTL", "Time to open (ms)"="Time to open (ms)", "Time to close (ms)"="Time to close (ms)") -> (w247:T7)
        n135 = local write "Exposições realizadas"(u8 0 ("Exposições realizadas")) -> ()
        n136 = Bundle By Name(cluster=w247, "Image Format"="Image Format", "Tiff Position"="Tiff Position", "Tiff Type"="Tiff Type", "Image Path"=w215) -> (w229:T7)
        n137 = call "Read RxTxCamera.lvclass.vi"("error in (no error)"=w228, "Application in"=w227) -> ("error out"=w231:errorcluster, "RxTxCamera.lvclass"=w232:refnum<class "RxTxCamera.lvclass">, "Application out"=w230:refnum<class "Application.lvclass">)  [unwired: 7 in]
        n138 = call "Write Config String.vi"("error in (no error)"=w231, "RED Channel Settings"=w229, "RxTxCamera in"=w232) -> ("error out"=w221:errorcluster, "RxTxCamera out"=w220:refnum<class "RxTxCamera.lvclass">)  [unwired: 7 in]
        n139 = call "Enqeue message.vi"("error in (no error)"=w221, "RxTx in"=w220) -> ("error out"=w218:errorcluster, "RxTx out"=w219:refnum<class "RxTxCamera.lvclass">)  [unwired: 8 in]
        n140 = call "Write RxTxCamera.lvclass.vi"("error in (no error)"=w218, "RxTxCamera.lvclass"=w219, "Application in"=w230) -> ("error out"=w226:errorcluster, "Application out"=w225:refnum<class "Application.lvclass">)  [unwired: 7 in]
        n141 = call "Read CCDCamera.lvclass.vi"("error in (no error)"=w226, "Application in"=w225) -> ("error out"=w223:errorcluster, "CCDCamera.lvclass"=w224:refnum<class "CCDCamera.lvclass">, "Application out"=w222:refnum<class "Application.lvclass">)  [unwired: 7 in]
        n142 = local read "Night Directory"() -> (w340:string)
        n143 = call "Read State Machine.lvclass.vi"("error in (no error)"=w223, "Instrument in"=w224) -> ("error out"=w381:errorcluster, "State Machine.lvclass"=w380:refnum<class "State Machine.lvclass">, "Instrument out"=w376:refnum<class "CCDCamera.lvclass">)  [unwired: 7 in]
        n144 = call "Next State.vi"("error in (no error)"=w381, "New_State"=u32 1, "State Machine in"=w380) -> ("error out"=w378:errorcluster, "State Machine out"=w377:refnum<class "State Machine.lvclass">)  [unwired: 7 in]
        n145 = call "Write State Machine.lvclass.vi"("error in (no error)"=w378, "State Machine.lvclass"=w377, "Instrument in"=w376) -> ("error out"=w375:errorcluster, "Instrument out"=w217:refnum<class "CCDCamera.lvclass">)  [unwired: 7 in]
        n146 = Bundle By Name(cluster=T15 {"Observer"="ECHARPE", "Object"="UNDEFINED", "Program ID"="UNDEFINED", "Night Directory"=""} ("User attributes"), "Observer"="Observer", "Object"="Object", "Program ID"="Program ID", "Night Directory"=w340) -> (w345:T15)
        n147 = call "Write CCDCamera.lvclass.vi"("error in (no error)"=w375, "CCDCamera.lvclass"=w217, "Application in"=w222) -> ("error out"=w352:errorcluster, "Application out"=w351:refnum<class "Application.lvclass">)  [unwired: 7 in]
        n148 = call "Read User.lvclass.vi"("error in (no error)"=w352, "Application in"=w351) -> ("error out"=w347:errorcluster, "User.lvclass"=w350:refnum<class "User.lvclass">, "Application out"=w346:refnum<class "Application.lvclass">)  [unwired: 7 in]
        n149 = local read "Sidereal Time"() -> (w332:string)
        n150 = local read "Air Mass"() -> (w237:string)
        n151 = call "Write User Attributes.vi"("error in (no error)"=w347, "User attributes"=w345, "User in"=w350) -> ("error out"=w348:errorcluster, "User out"=w349:refnum<class "User.lvclass">)  [unwired: 7 in]
        n152 = local read "Air Mass"() -> (w328:string)
        n153 = local read "Focus"() -> (w330:string)
        n154 = local read "HA"() -> (w238:string)
        n155 = local read "DEC"() -> (w240:string)
        n156 = local read "RA"() -> (w241:string)
        n157 = local read "UT"() -> (w331:string)
        n158 = local read "PA"() -> (w329:string)
        n159 = call "Write User.lvclass.vi"("error in (no error)"=w348, "User.lvclass"=w349, "Application in"=w346) -> ("error out"=w338:errorcluster, "Application out"=w339:refnum<class "Application.lvclass">)  [unwired: 7 in]
        n160 = Bundle By Name(cluster=T14 {"RA"="", "DEC"="", "TELRA"="", "TELDEC"="", "RA_DEG"="", "DEC_DEG"="", "Epoch"="", "AirMass"="", "Initial Air Mass"="", "HA"="", "HAD"="", "Final Air Mass"="", "X Offset"="", "Y Offset"="", "PA"="", "Camera Focus"="", "TCS Focus"="", "Moon distance"="", "Moon height"="", "Moon Phase"="", "TCSST"="", "TCSUT"=""} ("TCS Infos"), "RA"=w241, "DEC"=w240, "TELRA"=w241, "TELDEC"=w240, "RA_DEG"=w241, "DEC_DEG"=w240, "Epoch"="2000" ("AirMass"), "AirMass"=w328, "HA"=w238, "HAD"=w238) -> (w326:T14)
        n161 = Bundle By Name(cluster=w326, "Initial Air Mass"=w237, "Final Air Mass"=w237, "X Offset"=w236, "Y Offset"=w236, "PA"=w329, "Camera Focus"=w330, "TCS Focus"=w330, "Moon distance"=w235, "Moon height"=w235, "Moon Phase"="Crescente" ("AirMass"), "TCSUT"=w331, "TCSST"=w332) -> (w325:T14)
        n162 = call "Read TCS.lvclass.vi"("error in (no error)"=w338, "Application in"=w339) -> ("error out"=w336:errorcluster, "TCS.lvclass"=w337:refnum<class "TCS.lvclass">, "Application out"=w335:refnum<class "Application.lvclass">)  [unwired: 7 in]
        n163 = call "Write TCS Infos.vi"("error in (no error)"=w336, "TCS Infos"=w325, "TCS in"=w337) -> ("error out"=w333:errorcluster, "TCS out"=w334:refnum<class "TCS.lvclass">)  [unwired: 7 in]
        n164 = call "Write TCS.lvclass.vi"("error in (no error)"=w333, "TCS.lvclass"=w334, "Application in"=w335) -> ("error out"=w268:errorcluster, "Application out"=w267:refnum<class "Application.lvclass">)  [unwired: 7 in]
        n165 = case shown="\"1\"" "Read mode" {
          tunnel: ["NO SELECTION" "FAST" "NORMAL" "SLOW"] -> w320
          frame "No Selection", Default {
          }
          frame "1" {
          }
          frame "2" {
          }
          frame "3" {
          }
        }
        n166 = local read "Calibration Fiber"() -> (w243:bool)
        n167 = local read "Guiando"() -> (w309:bool)
        n168 = call "Read Observation type.vi"("error in (no error)"=w268, "Application in"=w267) -> ("error out"=w265:errorcluster, "Observation type"=w264:string, "Application out"=w266:refnum<class "Application.lvclass">)  [unwired: 7 in]
        n169 = local read "Sky Fiber"() -> (w242:bool)
        n170 = local read "Date"() -> (w323:string)
        n171 = case shown="True" w309 {
          tunnel: ["OFF" "ON"] -> w308
          frame False {
          }
          frame True {
          }
        }
        n172 = Bundle By Name(cluster=T13 {"Observation type"="", "Read Mode"="", "Sky fiber"=FALSE, "Calibration fiber"=FALSE, "Sync Mode"="", "Date"=""} ("Interface Infos"), "Observation type"=w264, "Read Mode"=w320, "Sky fiber"=w242, "Calibration fiber"=w243, "Date"=w323) -> (w322:T13)
        n173 = Bundle By Name(cluster=T11 {"THARLAMP"="", "HALLAMP"="", "AGITATOR"="", "THARMIRR"=""} ("Calibration Unit Contents"), "THARLAMP"=w296, "HALLAMP"=w296, "AGITATOR"=w296, "THARMIRR"="SPECTROGRAPH") -> (w305:T11)
        n174 = Bundle By Name(cluster=T12 {"GUIDING"="", "GUIDTEXP"="", "GUIDFREQ"="", "GUIDOBJX"="", "GUIDOBJY"="", "AVGYCOOR"="", "AVGXCORR"="", "GFOCUS"=""} ("Guider Contents"), "GUIDING"=w308, "GUIDTEXP"=w307, "GUIDFREQ"=w307, "GUIDOBJX"=w306, "GUIDOBJY"=w306, "AVGYCOOR"=w306, "AVGXCORR"=w306, "GFOCUS"=w306) -> (w316:T12)
        n175 = Bundle By Name(cluster=T10 {"TEMPEXT"="", "PRESSURE"="", "HUMIDITY"="", "WINDDIR"="", "WSPEED"=""} ("Weather Station Contents"), "TEMPEXT"="10.0", "PRESSURE"="742.00", "HUMIDITY"="92.00", "WINDDIR"="15.0", "WSPEED"="30.2") -> (w286:T10)
        n176 = call "Write Interface Infos.vi"("error in (no error)"=w265, "Interface Infos"=w322, "Application in"=w266) -> ("error out"=w318:errorcluster, "Application out"=w317:refnum<class "Application.lvclass">)  [unwired: 7 in]
        n177 = call "Read Guider.lvclass.vi"("error in (no error)"=w318, "Application in"=w317) -> ("error out"=w314:errorcluster, "Guider.lvclass"=w313:refnum<class "Guider.lvclass">, "Application out"=w312:refnum<class "Application.lvclass">)  [unwired: 7 in]
        n178 = call "Write Status.vi"("error in (no error)"=w314, "Guider Contents"=w316, "Guider in"=w313) -> ("error out"=w311:errorcluster, "Guider out"=w310:refnum<class "Guider.lvclass">)  [unwired: 7 in]
        n179 = call "Write Guider.lvclass.vi"("error in (no error)"=w311, "Guider.lvclass"=w310, "Application in"=w312) -> ("error out"=w303:errorcluster, "Application out"=w302:refnum<class "Application.lvclass">)  [unwired: 7 in]
        n180 = call "Read Calibration Unit.lvclass.vi"("error in (no error)"=w303, "Application in"=w302) -> ("error out"=w298:errorcluster, "Calibration Unit.lvclass"=w301:refnum<class "Calibration Unit.lvclass">, "Application out"=w299:refnum<class "Application.lvclass">)  [unwired: 7 in]
        n181 = call "Write Status.vi"("error in (no error)"=w298, "Calibration Unit Contents"=w305, "Calibration Unit in"=w301) -> ("error out"=w297:errorcluster, "Calibration Unit out"=w300:refnum<class "Calibration Unit.lvclass">)  [unwired: 7 in]
        n182 = call "Write Calibration Unit.lvclass.vi"("error in (no error)"=w297, "Calibration Unit.lvclass"=w300, "Application in"=w299) -> ("error out"=w289:errorcluster, "Application out"=w288:refnum<class "Application.lvclass">)  [unwired: 7 in]
        n183 = call "Read Weather Station.lvclass.vi"("error in (no error)"=w289, "Application in"=w288) -> ("error out"=w294:errorcluster, "Weather Station.lvclass"=w293:refnum<class "Weather Station.lvclass">, "Application out"=w291:refnum<class "Application.lvclass">)  [unwired: 7 in]
        n184 = call "Write Status.vi"("error in (no error)"=w294, "Weather Station Contents"=w286, "Weather Station in"=w293) -> ("error out"=w290:errorcluster, "Weather Station out"=w292:refnum<class "Weather Station.lvclass">)  [unwired: 7 in]
        n185 = call "Write Weather Station.lvclass.vi"("error in (no error)"=w290, "Weather Station.lvclass"=w292, "Application in"=w291) -> ("error out"=w280:errorcluster, "Application out"=w279:refnum<class "Application.lvclass">)  [unwired: 7 in]
        n186 = Bundle By Name(cluster=T9 {"ADC"="", "ADCSPEED"="", "CALMIRR"=""} ("Fore Optics Contents"), "ADC"="ON", "ADCSPEED"="5.0", "CALMIRR"="OUT") -> (w275:T9)
        n187 = Bundle By Name(cluster=T8 {"DSTATUS"="", "DPOS"="", "DTEMP"="", "DHUM"="", "DLAMP"="", "DFLAT"=""} ("Dome Contents"), "DSTATUS"="OPEN", "DPOS"="0.00000", "DTEMP"="10", "DHUM"="82.0", "DLAMP"=w252, "DFLAT"=w252) -> (w253:T8)
        n188 = call "Read Fore Optics.lvclass.vi"("error in (no error)"=w280, "Application in"=w279) -> ("error out"=w278:errorcluster, "Fore Optics.lvclass"=w277:refnum<class "Fore Optics.lvclass">, "Application out"=w272:refnum<class "Application.lvclass">)  [unwired: 7 in]
        n189 = call "Write Status.vi"("error in (no error)"=w278, "Fore Optics Contents"=w275, "Fore Optics in"=w277) -> ("error out"=w274:errorcluster, "Fore Optics out"=w273:refnum<class "Fore Optics.lvclass">)  [unwired: 7 in]
        n190 = call "Write Fore Optics.lvclass.vi"("error in (no error)"=w274, "Fore Optics.lvclass"=w273, "Application in"=w272) -> ("error out"=w261:errorcluster, "Application out"=w260:refnum<class "Application.lvclass">)  [unwired: 7 in]
        n191 = call "Read Dome.lvclass.vi"("error in (no error)"=w261, "Application in"=w260) -> ("error out"=w255:errorcluster, "Dome.lvclass"=w256:refnum<class "Dome.lvclass">, "Application out"=w257:refnum<class "Application.lvclass">)  [unwired: 7 in]
        n192 = call "Write Status.vi"("error in (no error)"=w255, "Dome Contents"=w253, "Dome in"=w256) -> ("error out"=w259:errorcluster, "Dome out"=w258:refnum<class "Dome.lvclass">)  [unwired: 7 in]
        n193 = call "Write Dome.lvclass.vi"("error in (no error)"=w259, "Dome.lvclass"=w258, "Application in"=w257) -> ("error out"=w263:errorcluster, "Application out"=w262:refnum<class "Application.lvclass">)  [unwired: 7 in]
      }
      event "Read mode": Value Change {
        # "Esta operação carrega na interface as informações relativas à pré-configuração de fast, normal ou slow acquisitions"
        n194 = event-data() -> ()  [unwired: 1 in, 1 out]
        n195 = local read "Read mode"() -> (w404:enum32{"No Selection", "1", "2", "3"})
        n196 = call "Read Setup File.lvclass.vi"("error in (no error)"=w403, "Application in"=w402) -> ("error out"=w397:errorcluster, "Setup File.lvclass"=w398:refnum<class "Setup File.lvclass">, "Application out"=w401:refnum<class "Application.lvclass">)  [unwired: 7 in]
        n197 = case shown="\"1\"" w404 {
          tunnel: [_ "Fast.txt" "Normal.txt" "Slow.txt"] -> w396
          frame "No Selection", Default {
          }
          frame "1" {
          }
          frame "2" {
          }
          frame "3" {
          }
        }
        n198 = call "Write File Name.vi"("error in (no error)"=w397, "File Name"=w396, "Setup File in"=w398) -> ("error out"=w400:errorcluster, "Setup File out"=w399:refnum<class "Setup File.lvclass">)  [unwired: 7 in]
        n199 = call "Read File.vi"("error in (no error)"=w400, "Setup File in"=w399) -> ("error out"=w392:errorcluster, "Setup"=w395:T16, "Setup File out"=w391:refnum<class "Setup File.lvclass">)  [unwired: 7 in]
        n200 = call "Read File Path.vi"("error in (no error)"=w392, "Setup File in"=w391) -> ("error out"=w389:errorcluster, "File Path"=w388:string, "Setup File out"=w390:refnum<class "Setup File.lvclass">)  [unwired: 7 in]
        n201 = stacked-sequence {
          tunnel: w395 -> [w409 w421]
          frame #0 {
            n202 = Unbundle By Name(w409) -> ("VShift Speed"=w406:string)
            n203 = To Upper Case(1:w406) -> (0:w410:string)
            n204 = Concatenate Strings("Invalid VShift Speed value: ", w406) -> (w405:string)
            n205 = case shown="\"False\", Default" w410 {
              tunnel: [_ w413 w414 w415 w416] -> w408
              tunnel: w405 -> [w411 _ _ _ _]
              frame "False", Default {
                n206 = One Button Dialog(message=w411, button name ("OK")="OK") -> ()  [unwired: 1 out]
              }
              frame "2.2" {
                w413 = u8 1 items=["0.6", "2.2", "3.6", "4.33"] ("Vertical Shift Speed")
              }
              frame "3.6" {
                w414 = u8 2 items=["0.6", "2.2", "3.6", "4.33"] ("Vertical Shift Speed")
              }
              frame "4.33" {
                w415 = u8 3 items=["0.6", "2.2", "3.6", "4.33"] ("Vertical Shift Speed")
              }
              frame "0.6" {
                w416 = u8 0 items=["0.6", "2.2", "3.6", "4.33"] ("Vertical Shift Speed")
              }
            }
            n207 = local write "Vertical Shift Speed"(w408) -> ()
          }
          frame #1 {
            n208 = Unbundle By Name(w421) -> ("Readout rate"=w418:string)
            n209 = Concatenate Strings("Invalid Readout Rate value: ", w418) -> (w417:string)
            n210 = To Upper Case(1:w418) -> (0:w422:string)
            n211 = case shown="\"False\", Default" w422 {
              tunnel: [_ w425 w426] -> w420
              tunnel: w417 -> [w423 _ _]
              frame "False", Default {
                n212 = One Button Dialog(message=w423, button name ("OK")="OK") -> ()  [unwired: 1 out]
              }
              frame "1MHZAT16BIT" {
                w425 = u8 1 items=["100 KHz at 16 bit", "1 MHz at 16 bit"] ("Readout Rate")
              }
              frame "100KHZAT16BIT" {
                w426 = u8 0 items=["100 KHz at 16 bit", "1 MHz at 16 bit"] ("Readout Rate")
              }
            }
            n213 = local write "Readout Rate"(w420) -> ()
          }
        }
        n214 = call "Write Setup File.lvclass.vi"("error in (no error)"=w389, "Setup File.lvclass"=w390, "Application in"=w401) -> ("error out"=w394:errorcluster, "Application out"=w393:refnum<class "Application.lvclass">)  [unwired: 7 in]
        n215 = local write "Setup File Path:"(w388) -> ()
      }
      event "Load Setup", "Load Seup 2": Value Change {
        # "Esta operação irá carregar na interface as informações do modo de operação da câmera contidas num arquivo texto fornecido pelo usuário."
        n216 = event-data() -> ()  [unwired: 1 in, 1 out]
        n217 = call "File Dialog"() -> ("selected path"=w440:path)  [unwired: 12 in, 3 out]
        n218 = call "Read Setup File.lvclass.vi"("error in (no error)"=w445, "Application in"=w444) -> ("error out"=w441:errorcluster, "Setup File.lvclass"=w442:refnum<class "Setup File.lvclass">, "Application out"=w447:refnum<class "Application.lvclass">)  [unwired: 7 in]
        n219 = call "Select File.vi"("error in (no error)"=w441, "File Path Control"=w440, "Setup File in"=w442) -> ("error out"=w434:errorcluster, "Setup File out"=w433:refnum<class "Setup File.lvclass">)  [unwired: 7 in]
        n220 = call "Read File Path.vi"("error in (no error)"=w434, "Setup File in"=w433) -> ("error out"=w430:errorcluster, "File Path"=→"Setup File Path:":string, "Setup File out"=w431:refnum<class "Setup File.lvclass">)  [unwired: 7 in]
        n221 = call "Read File.vi"("error in (no error)"=w430, "Setup File in"=w431) -> ("error out"=w446:errorcluster, "Setup"=w443:T16, "Setup File out"=w448:refnum<class "Setup File.lvclass">)  [unwired: 7 in]
        n222 = call "Write Setup File.lvclass.vi"("error in (no error)"=w446, "Setup File.lvclass"=w448, "Application in"=w447) -> ("error out"=w437:errorcluster, "Application out"=w439:refnum<class "Application.lvclass">)  [unwired: 7 in]
        n223 = call "Read CCDCamera.lvclass.vi"("error in (no error)"=w437, "Application in"=w439) -> ("error out"=w436:errorcluster, "CCDCamera.lvclass"=w435:refnum<class "CCDCamera.lvclass">, "Application out"=w438:refnum<class "Application.lvclass">)  [unwired: 7 in]
        n224 = stacked-sequence {
          tunnel: w443 -> [w453 w468 w484 w496 w512 w524 w534 w545 w556 w571 w609 w646 w689]
          tunnel: w435 -> [_ _ _ _ _ _ _ _ _ _ _ w645 _]
          frame #0 {
            n225 = Unbundle By Name(w453) -> ("Acquisition Mode"=w450:string)
            n226 = To Upper Case(1:w450) -> (0:w454:string)
            n227 = Concatenate Strings("Invalid Aquisition Mode value: ", w450) -> (w449:string)
            n228 = case shown="\"\"" w454 {
              tunnel: [_ _ w457 w458 w459 w460 w461 w462 w463] -> w452
              tunnel: w449 -> [w456 _ _ _ _ _ _ _ _]
              frame "False", Default {
                n229 = One Button Dialog(message=w456, button name ("OK")="OK") -> ()  [unwired: 1 out]
              }
              frame "" {
              }
              frame "RESERVED" {
                w457 = u16 0 items=["RESERVED", "Single Scan", "Accumulate", "Kinetics", "Fast Kinetics", "Run Til Abort", "RESERVED", "RESERVED", "RESERVED", "RESERVED", "Time Delayed Integration"] ("Acquisition Mode")
              }
              frame "SINGLE" {
                w458 = u16 1 items=["RESERVED", "Single Scan", "Accumulate", "Kinetics", "Fast Kinetics", "Run Til Abort", "RESERVED", "RESERVED", "RESERVED", "RESERVED", "Time Delayed Integration"] ("Acquisition Mode")
              }
              frame "ACCUMULATE" {
                w459 = u16 2 items=["RESERVED", "Single Scan", "Accumulate", "Kinetics", "Fast Kinetics", "Run Til Abort", "RESERVED", "RESERVED", "RESERVED", "RESERVED", "Time Delayed Integration"] ("Acquisition Mode")
              }
              frame "KINETICS" {
                w460 = u16 3 items=["RESERVED", "Single Scan", "Accumulate", "Kinetics", "Fast Kinetics", "Run Til Abort", "RESERVED", "RESERVED", "RESERVED", "RESERVED", "Time Delayed Integration"] ("Acquisition Mode")
              }
              frame "FASTKINETICS" {
                w461 = u16 4 items=["RESERVED", "Single Scan", "Accumulate", "Kinetics", "Fast Kinetics", "Run Til Abort", "RESERVED", "RESERVED", "RESERVED", "RESERVED", "Time Delayed Integration"] ("Acquisition Mode")
              }
              frame "RUNTILABORT" {
                w462 = u16 4 items=["RESERVED", "Single Scan", "Accumulate", "Kinetics", "Fast Kinetics", "Run Til Abort", "RESERVED", "RESERVED", "RESERVED", "RESERVED", "Time Delayed Integration"] ("Acquisition Mode")
              }
              frame "TIMEDELAYEDINTEGRATION" {
                w463 = u16 10 items=["RESERVED", "Single Scan", "Accumulate", "Kinetics", "Fast Kinetics", "Run Til Abort", "RESERVED", "RESERVED", "RESERVED", "RESERVED", "Time Delayed Integration"] ("Acquisition Mode")
              }
            }
            n230 = local write "Acquisition Mode"(w452) -> ()
          }
          frame #1 {
            n231 = Unbundle By Name(w468) -> ("Trigger"=w465:string)
            n232 = To Upper Case(1:w465) -> (0:w469:string)
            n233 = Concatenate Strings("Invalid Trigger value: ", w465) -> (w464:string)
            n234 = case shown="\"\"" w469 {
              tunnel: [_ _ w472 w473 w474 w475 w476 w477 w478 w479] -> w467
              tunnel: w464 -> [w470 _ _ _ _ _ _ _ _ _]
              frame "False", Default {
                n235 = One Button Dialog(message=w470, button name ("OK")="OK") -> ()  [unwired: 1 out]
              }
              frame "" {
              }
              frame "N/A" {
                w472 = u16 2 items=["Internal", "External", "N/A", "N/A", "N/A", "N/A", "External Start", "External Exposure (bulb)", "N/A", "External FVB EM", "Software", "N/A", "External Charge Shifting"] ("Trigger")
              }
              frame "EXTERNALSTART" {
                w473 = u16 6 items=["Internal", "External", "N/A", "N/A", "N/A", "N/A", "External Start", "External Exposure (bulb)", "N/A", "External FVB EM", "Software", "N/A", "External Charge Shifting"] ("Trigger")
              }
              frame "EXTERNALEXPOSURE(BULB)" {
                w474 = u16 7 items=["Internal", "External", "N/A", "N/A", "N/A", "N/A", "External Start", "External Exposure (bulb)", "N/A", "External FVB EM", "Software", "N/A", "External Charge Shifting"] ("Trigger")
              }
              frame "EXTERNALFVBEM" {
                w475 = u16 9 items=["Internal", "External", "N/A", "N/A", "N/A", "N/A", "External Start", "External Exposure (bulb)", "N/A", "External FVB EM", "Software", "N/A", "External Charge Shifting"] ("Trigger")
              }
              frame "SOFTWARE" {
                w476 = u16 10 items=["Internal", "External", "N/A", "N/A", "N/A", "N/A", "External Start", "External Exposure (bulb)", "N/A", "External FVB EM", "Software", "N/A", "External Charge Shifting"] ("Trigger")
              }
              frame "EXTERNALCHARGESHIFTING" {
                w477 = u16 12 items=["Internal", "External", "N/A", "N/A", "N/A", "N/A", "External Start", "External Exposure (bulb)", "N/A", "External FVB EM", "Software", "N/A", "External Charge Shifting"] ("Trigger")
              }
              frame "INTERNAL" {
                w478 = u16 0 items=["Internal", "External", "N/A", "N/A", "N/A", "N/A", "External Start", "External Exposure (bulb)", "N/A", "External FVB EM", "Software", "N/A", "External Charge Shifting"] ("Trigger")
              }
              frame "EXTERNAL" {
                w479 = u16 1 items=["Internal", "External", "N/A", "N/A", "N/A", "N/A", "External Start", "External Exposure (bulb)", "N/A", "External FVB EM", "Software", "N/A", "External Charge Shifting"] ("Trigger")
              }
            }
            n236 = local write "Trigger"(w467) -> ()
          }
          frame #2 {
            n237 = Unbundle By Name(w484) -> ("Read Mode"=w481:string)
            n238 = To Upper Case(1:w481) -> (0:w485:string)
            n239 = Concatenate Strings("Invalid Read Mode value: ", w481) -> (w480:string)
            n240 = case shown="\"\"" w485 {
              tunnel: [_ _ w488 w489 w490 w491 w492] -> w483
              tunnel: w480 -> [w486 _ _ _ _ _ _]
              frame "False", Default {
                n241 = One Button Dialog(message=w486, button name ("OK")="OK") -> ()  [unwired: 1 out]
              }
              frame "" {
              }
              frame "FULLVERTICALBINNING " {
                w488 = u16 0 items=["Full Vertical Binning", "Multi-Track", "Random-Track", "Single-Track", "Image"] ("Read Mode")
              }
              frame "MULTI-TRACK" {
                w489 = u16 1 items=["Full Vertical Binning", "Multi-Track", "Random-Track", "Single-Track", "Image"] ("Read Mode")
              }
              frame "RANDOM-TRACK" {
                w490 = u16 2 items=["Full Vertical Binning", "Multi-Track", "Random-Track", "Single-Track", "Image"] ("Read Mode")
              }
              frame "SINGLE-TRACK" {
                w491 = u16 3 items=["Full Vertical Binning", "Multi-Track", "Random-Track", "Single-Track", "Image"] ("Read Mode")
              }
              frame "IMAGE" {
                w492 = u16 4 items=["Full Vertical Binning", "Multi-Track", "Random-Track", "Single-Track", "Image"] ("Read Mode")
              }
            }
            n242 = local write "Read Mode"(w483) -> ()
          }
          frame #3 {
            n243 = Unbundle By Name(w496) -> ("Exposure Time"=w493:string)
            n244 = Not Equal?(x="", y=w493) -> (x != y?=w494:bool)
            n245 = case shown="True" w494 {
              tunnel: w493 -> [_ w498]
              frame False {
              }
              frame True {
                n246 = Fract/Exp String To Number(string=w498) -> (number=w497:dbl)  [unwired: 3 in, 1 out]
                n247 = Less?(x=w497, y=0.0) -> (x < y?=w499:bool)
                n248 = case shown="False" w499 {
                  tunnel: w497 -> [w502 w505]
                  tunnel: "Exposure time lower than zero: " -> [_ w503]
                  frame False {
                    n249 = local write "Exposure time"(w502) -> ()
                    n250 = local write "Exposure Time (s)  2"(w502) -> ()
                  }
                  frame True {
                    n251 = Number To Fractional String(number=w505) -> (F-format string=w504:string)  [unwired: 3 in]
                    n252 = Concatenate Strings(w503, w504) -> (w506:string)
                    n253 = One Button Dialog(message=w506, button name ("OK")="OK") -> ()  [unwired: 1 out]
                  }
                }
              }
            }
          }
          frame #4 {
            n254 = Unbundle By Name(w512) -> ("VShift Speed"=w509:string)
            n255 = To Upper Case(1:w509) -> (0:w513:string)
            n256 = Concatenate Strings("Invalid VShift Speed value: ", w509) -> (w508:string)
            n257 = case shown="\"\"" w513 {
              tunnel: [_ _ w516 w517 w518 w519] -> w511
              tunnel: w508 -> [w514 _ _ _ _ _]
              frame "False", Default {
                n258 = One Button Dialog(message=w514, button name ("OK")="OK") -> ()  [unwired: 1 out]
              }
              frame "" {
              }
              frame "2.2" {
                w516 = u8 1 items=["0.6", "2.2", "3.6", "4.33"] ("Vertical Shift Speed")
              }
              frame "3.6" {
                w517 = u8 2 items=["0.6", "2.2", "3.6", "4.33"] ("Vertical Shift Speed")
              }
              frame "4.33" {
                w518 = u8 3 items=["0.6", "2.2", "3.6", "4.33"] ("Vertical Shift Speed")
              }
              frame "0.6" {
                w519 = u8 0 items=["0.6", "2.2", "3.6", "4.33"] ("Vertical Shift Speed")
              }
            }
            n259 = local write "Vertical Shift Speed"(w511) -> ()
          }
          frame #5 {
            n260 = Unbundle By Name(w524) -> ("Readout rate"=w521:string)
            n261 = Concatenate Strings("Invalid Readout Rate value: ", w521) -> (w520:string)
            n262 = To Upper Case(1:w521) -> (0:w525:string)
            n263 = case shown="\"\"" w525 {
              tunnel: [_ _ w528 w529] -> w523
              tunnel: w520 -> [w526 _ _ _]
              frame "False", Default {
                n264 = One Button Dialog(message=w526, button name ("OK")="OK") -> ()  [unwired: 1 out]
              }
              frame "" {
              }
              frame "1MHZAT16BIT" {
                w528 = u8 1 items=["100 KHz at 16 bit", "1 MHz at 16 bit"] ("Readout Rate")
              }
              frame "100KHZAT16BIT" {
                w529 = u8 0 items=["100 KHz at 16 bit", "1 MHz at 16 bit"] ("Readout Rate")
              }
            }
            n265 = local write "Readout Rate"(w523) -> ()
          }
          frame #6 {
            n266 = Unbundle By Name(w534) -> ("Pre amp"=w531:string)
            n267 = Concatenate Strings("Invalid Pre-amp value: ", w531) -> (w530:string)
            n268 = To Upper Case(1:w531) -> (0:w535:string)
            n269 = case shown="\"\"" w535 {
              tunnel: [_ _ w538 w539 w540] -> w533
              tunnel: w530 -> [w536 _ _ _ _]
              frame "False", Default {
                n270 = One Button Dialog(message=w536, button name ("OK")="OK") -> ()  [unwired: 1 out]
              }
              frame "" {
              }
              frame "1" {
                w538 = u8 0 items=["1", "2", "4"] ("Pre-amplifier gain")
              }
              frame "2" {
                w539 = u8 1 items=["1", "2", "4"] ("Pre-amplifier gain")
              }
              frame "4" {
                w540 = u8 2 items=["1", "2", "4"] ("Pre-amplifier gain")
              }
            }
            n271 = local write "Pre-amplifier gain"(w533) -> ()
          }
          frame #7 {
            n272 = Unbundle By Name(w545) -> ("Shutter Mode"=w543:string)
            n273 = Concatenate Strings("Invalid Shutter Mode value: ", w543) -> (w541:string)
            n274 = To Upper Case(1:w543) -> (0:w546:string)
            n275 = case shown="\"\"" w546 {
              tunnel: [_ _ w549 w550 w551] -> w544
              tunnel: w541 -> [w547 _ _ _ _]
              frame "False", Default {
                n276 = One Button Dialog(message=w547, button name ("OK")="OK") -> ()  [unwired: 1 out]
              }
              frame "" {
              }
              frame "FULLYAUTO" {
                w549 = u16 0 items=["Fully Auto", "OPEN", "CLOSED"] ("Shutter Mode")
              }
              frame "OPEN" {
                w550 = u16 1 items=["Fully Auto", "OPEN", "CLOSED"] ("Shutter Mode")
              }
              frame "CLOSED" {
                w551 = u16 2 items=["Fully Auto", "OPEN", "CLOSED"] ("Shutter Mode")
              }
            }
            n277 = local write "Shutter Mode"(w544) -> ()
          }
          frame #8 {
            n278 = Unbundle By Name(w556) -> ("Shutter TTL"=w553:string)
            n279 = To Upper Case(1:w553) -> (0:w557:string)
            n280 = Concatenate Strings("Invalid Shutter TTL value: ", w553) -> (w552:string)
            n281 = case shown="\"\"" w557 {
              tunnel: [_ _ w560 w561] -> w555
              tunnel: w552 -> [w558 _ _ _]
              frame "False", Default {
                n282 = One Button Dialog(message=w558, button name ("OK")="OK") -> ()  [unwired: 1 out]
              }
              frame "" {
              }
              frame "TTLHIGH" {
                w560 = u16 1 items=["TTL Low", "TTL High"] ("Shutter TTL")
              }
              frame "TTLLOW" {
                w561 = u16 0 items=["TTL Low", "TTL High"] ("Shutter TTL")
              }
            }
            n283 = local write "Shutter TTL"(w555) -> ()
          }
          frame #9 {
            n284 = Unbundle By Name(w571) -> ("Time to open shutter"=w568:string, "Time to close shutter"=w565:string, "Temperature"=w562:string)
            n285 = Not Equal?(x="", y=w562) -> (x != y?=w563:bool)
            n286 = case shown="True" w563 {
              tunnel: w562 -> [_ w572]
              frame False {
              }
              frame True {
                n287 = property on="Set temperature" class="DigNum (strict)"() -> ("Maximum"=w578:dbl)  [unwired: 2 in, 2 out]
                n288 = property on="Set temperature" class="DigNum (strict)"() -> ("Minimum"=w577:dbl)  [unwired: 2 in, 2 out]
                n289 = Decimal String To Number(string=w572) -> (number=w573:i32)  [unwired: 2 in, 1 out]
                n290 = Greater?(x=w573, y=w578) -> (0:w575:bool)
                n291 = Less?(x=w573, y=w577) -> (x < y?=w576:bool)
                n292 = Or(x=w575, y=w576) -> (x .or. y?=w574:bool)
                n293 = case shown="False" w574 {
                  tunnel: w573 -> [w579 w580]
                  frame False {
                    n294 = local write "Set temperature"(w579) -> ()
                  }
                  frame True {
                    n295 = Number To Decimal String(number=w580) -> (decimal integer string=w581:string)  [unwired: 1 in]
                    n296 = Concatenate Strings("Temperature value outside allowed range: ", w581) -> (w583:string)
                    n297 = One Button Dialog(message=w583, button name ("OK")="OK") -> ()  [unwired: 1 out]
                  }
                }
              }
            }
            n298 = Not Equal?(x="", y=w565) -> (x != y?=w567:bool)
            n299 = Not Equal?(x="", y=w568) -> (x != y?=w570:bool)
            n300 = case shown="True" w567 {
              tunnel: w565 -> [_ w585]
              frame False {
              }
              frame True {
                n301 = Decimal String To Number(string=w585) -> (number=w586:i32)  [unwired: 2 in, 1 out]
                n302 = Less?(x=w586, y=50) -> (x < y?=w587:bool)
                n303 = case shown="False" w587 {
                  tunnel: w586 -> [w589 w590]
                  frame False {
                    n304 = local write "Time to close (ms)"(w589) -> ()
                  }
                  frame True {
                    n305 = Number To Decimal String(number=w590) -> (decimal integer string=w591:string)  [unwired: 1 in]
                    n306 = Concatenate Strings("Time to close shutter is lower than 50 ms: ", w591) -> (w593:string)
                    n307 = One Button Dialog(message=w593, button name ("OK")="OK") -> ()  [unwired: 1 out]
                  }
                }
              }
            }
            n308 = case shown="True" w570 {
              tunnel: w568 -> [_ w595]
              frame False {
              }
              frame True {
                n309 = Decimal String To Number(string=w595) -> (number=w596:i32)  [unwired: 2 in, 1 out]
                n310 = Less?(x=w596, y=50) -> (x < y?=w597:bool)
                n311 = case shown="False" w597 {
                  tunnel: w596 -> [w599 w600]
                  frame False {
                    n312 = local write "Time to open (ms)"(w599) -> ()
                  }
                  frame True {
                    n313 = Number To Decimal String(number=w600) -> (decimal integer string=w601:string)  [unwired: 1 in]
                    n314 = Concatenate Strings("Time to open shutter is lower than 50 ms: ", w601) -> (w603:string)
                    n315 = One Button Dialog(message=w603, button name ("OK")="OK") -> ()  [unwired: 1 out]
                  }
                }
              }
            }
          }
          frame #10 {
            n316 = Unbundle By Name(w609) -> ("Cooler"=w606:string)
            n317 = To Upper Case(1:w606) -> (0:w610:string)
            n318 = Concatenate Strings("Invalid Cooler value: ", w606) -> (w605:string)
            n319 = case shown="\"False\", Default" w610 {
              tunnel: [_ _ w613 w614] -> w608
              tunnel: w605 -> [w611 _ _ _]
              frame "False", Default {
                n320 = One Button Dialog(message=w611, button name ("OK")="OK") -> ()  [unwired: 1 out]
              }
              frame "" {
              }
              frame "OFF" {
                w613 = u16 0 items=["Cooler OFF", "Cooler ON"] ("Cooler ON/OFF")
              }
              frame "ON" {
                w614 = u16 1 items=["Cooler OFF", "Cooler ON"] ("Cooler ON/OFF")
              }
            }
            n321 = local write "Cooler ON/OFF"(w608) -> ()
          }
          frame #11 {
            w621 = i32[] [1, 2, 4, 8, 16, 32, 64]
            n322 = Unbundle By Name(w646) -> ("Initial Line"=w647:string, "Initial Column"=w639:string, "Final Line"=w635:string, "Final Column"=w631:string, "Horizontal binning"=w629:string, "Vertical binning"=w622:string)
            n323 = call "Read X lenght.vi"("CCDCamera in"=w645) -> ("X lenght"=w618:u16)  [unwired: 8 in, 2 out]
            n324 = call "Read Y lenght.vi"("CCDCamera in"=w645) -> ("Y lenght"=w616:u16)  [unwired: 8 in, 2 out]
            n325 = Increment(x=w618) -> (x+1=w617:u16)
            n326 = Increment(x=w616) -> (x+1=w615:u16)
            n327 = Decimal String To Number(string=w622) -> (number=w619:i32)  [unwired: 2 in, 1 out]
            n328 = Decimal String To Number(string=w629) -> (offset past number=w625:i32)  [unwired: 2 in, 1 out]
            n329 = Decimal String To Number(string=w647) -> (number=w643:i32)  [unwired: 2 in, 1 out]
            n330 = Decimal String To Number(string=w639) -> (number=w638:i32)  [unwired: 2 in, 1 out]
            n331 = Decimal String To Number(string=w635) -> (number=w634:i32)  [unwired: 2 in, 1 out]
            n332 = Equal?(x=w619, y=w621) -> (x = y?=w624:bool[])
            n333 = Decimal String To Number(string=w631) -> (number=w630:i32)  [unwired: 2 in, 1 out]
            n334 = Equal?(x=w625, y=w621) -> (x = y?=w628:bool[])
            n335 = Boolean To (0,1)(Boolean=w624) -> (0, 1=w620:i16[])
            n336 = Boolean To (0,1)(Boolean=w628) -> (0, 1=w627:i16[])
            n337 = Add Array Elements(numeric array=w620) -> (sum=w623:i16)
            n338 = In Range and Coerce(upper limit=w617, x=w630, lower limit=u16 0) -> (In Range?=w633:bool)  [unwired: 1 out]
            n339 = In Range and Coerce(upper limit=w615, x=w634, lower limit=u16 0) -> (In Range?=w637:bool)  [unwired: 1 out]
            n340 = Add Array Elements(numeric array=w627) -> (sum=w626:i16)
            n341 = In Range and Coerce(upper limit=w617, x=w638, lower limit=u16 0) -> (In Range?=w642:bool)  [unwired: 1 out]
            n342 = In Range and Coerce(upper limit=w615, x=w643, lower limit=0) -> (In Range?=w644:bool)  [unwired: 1 out]
            n343 = case shown="True" w637 {
              tunnel: w634 -> [w666 w671]
              frame False {
                n344 = Number To Decimal String(number=w666) -> (decimal integer string=w669:string)  [unwired: 1 in]
                n345 = Concatenate Strings("Final line outside allowed range: ", w669) -> (w668:string)
                n346 = One Button Dialog(message=w668, button name ("OK")="OK") -> ()  [unwired: 1 out]
              }
              frame True {
                n347 = local write "Final Line"(w671) -> ()
              }
            }
            n348 = case shown="0, Default" w626 {
              tunnel: w625 -> [w654 w659]
              frame 0, Default {
                n349 = Number To Decimal String(number=w654) -> (decimal integer string=w657:string)  [unwired: 1 in]
                n350 = Concatenate Strings("Invalid value for Horizontal Binning: ", w657) -> (w656:string)
                n351 = One Button Dialog(message=w656, button name ("OK")="OK") -> ()  [unwired: 1 out]
              }
              frame 1 {
                n352 = local write "Horizontal binning"(w659) -> ()
              }
            }
            n353 = case shown="False" w633 {
              tunnel: w630 -> [w660 w665]
              frame False {
                n354 = Number To Decimal String(number=w660) -> (decimal integer string=w663:string)  [unwired: 1 in]
                n355 = Concatenate Strings("Final column outside allowed range: ", w663) -> (w662:string)
                n356 = One Button Dialog(message=w662, button name ("OK")="OK") -> ()  [unwired: 1 out]
              }
              frame True {
                n357 = local write "Final Column"(w665) -> ()
              }
            }
            n358 = case shown="0, Default" w623 {
              selector: w623 -> [_ w653]
              tunnel: w619 -> [w648 _]
              frame 0, Default {
                n359 = Number To Decimal String(number=w648) -> (decimal integer string=w651:string)  [unwired: 1 in]
                n360 = Concatenate Strings("Invalid value for Vertical Binning: ", w651) -> (w650:string)
                n361 = One Button Dialog(message=w650, button name ("OK")="OK") -> ()  [unwired: 1 out]
              }
              frame 1 {
                n362 = local write "Vertical binning"(w653) -> ()
              }
            }
            n363 = case shown="True" w644 {
              tunnel: w643 -> [w680 w683]
              frame False {
                n364 = Number To Decimal String(number=w680) -> (decimal integer string=w681:string)  [unwired: 1 in]
                n365 = Concatenate Strings("Initial line outside allowed range: ", w681) -> (w679:string)
                n366 = One Button Dialog(message=w679, button name ("OK")="OK") -> ()  [unwired: 1 out]
              }
              frame True {
                n367 = local write "Initial Line"(w683) -> ()
              }
            }
            n368 = case shown="False" w642 {
              tunnel: w638 -> [w672 w677]
              frame False {
                n369 = Number To Decimal String(number=w672) -> (decimal integer string=w675:string)  [unwired: 1 in]
                n370 = Concatenate Strings("Initial column outside allowed range: ", w675) -> (w674:string)
                n371 = One Button Dialog(message=w674, button name ("OK")="OK") -> ()  [unwired: 1 out]
              }
              frame True {
                n372 = local write "Initial Column"(w677) -> ()
              }
            }
          }
          frame #12 {
            n373 = Unbundle By Name(w689) -> ("Sub image"=w685:string)
            n374 = Concatenate Strings("Invalid Sub Image value: ", w685) -> (w684:string)
            n375 = To Upper Case(1:w685) -> (0:w687:string)
            n376 = case shown="\"\"" w687 {
              tunnel: [_ _ T3."64 x 64" ("Sub Image") T3."128 x 128" ("Sub Image") T3."256 x 256" ("Sub Image") T3."512 x 512" ("Sub Image") T3."1024 x 1024" ("Sub Image") T3."Custom" ("Sub Image")] -> w688
              tunnel: w684 -> [w690 _ _ _ _ _ _ _]
              frame "False", Default {
                n377 = One Button Dialog(message=w690, button name ("OK")="OK") -> ()  [unwired: 1 out]
              }
              frame "" {
              }
              frame "64X64" {
              }
              frame "128X128" {
              }
              frame "256X256" {
              }
              frame "512X512" {
              }
              frame "1024X1024" {
              }
              frame "CUSTOM" {
              }
            }
            n378 = local write "Sub Image"(w688) -> ()
          }
        }
      }
      event "Save Setup": Value Change {
        # "Esta operação é responsável por reunir todas as informações da configuração do CCD da interface e escrevê-las em um arquivo texto"
        n379 = event-data() -> ()  [unwired: 1 in, 1 out]
        n380 = local read "Acquisition Mode"() -> (w749:u16)
        n381 = call "Read Setup File.lvclass.vi"("error in (no error)"=w751, "Application in"=w750) -> ("error out"=w712:errorcluster, "Setup File.lvclass"=w713:refnum<class "Setup File.lvclass">, "Application out"=w707:refnum<class "Application.lvclass">)  [unwired: 7 in]
        n382 = local read "Readout Rate"() -> (w741:u8)
        n383 = local read "Vertical Shift Speed"() -> (w739:u8)
        n384 = local read "Read Mode"() -> (w743:u16)
        n385 = local read "Shutter Mode"() -> (w735:u16)
        n386 = local read "Trigger"() -> (w747:u16)
        n387 = local read "Shutter TTL"() -> (w733:u16)
        n388 = local read "Pre-amplifier gain"() -> (w737:u8)
        n389 = case shown="1" w741 {
          tunnel: ["100 KHz at 16 bit" "1 MHz at 16 bit"] -> w740
          frame 0, Default {
          }
          frame 1 {
          }
        }
        n390 = case shown="9" w749 {
          tunnel: ["RESERVED" "Single" "Accumulate" "Kinetics" "Fast Kinetics" "Run Til Abort" "RESERVED" "RESERVED" "RESERVED" "Time Delayed Integration"] -> w748
          frame 0, Default {
          }
          frame 1 {
          }
          frame 2 {
          }
          frame 3 {
          }
          frame 4 {
          }
          frame 5 {
          }
          frame 6 {
          }
          frame 7 {
          }
          frame 8 {
          }
          frame 9 {
          }
        }
        n391 = case shown="12" w747 {
          tunnel: ["External" "N/A" "N/A" "N/A" "N/A" "External Start" "External Exposure (bulb)" "N/A" "External FVB EM" "Software" "N/A" "External Charge Shifting" "Internal"] -> w746
          frame 1 {
          }
          frame 2 {
          }
          frame 3 {
          }
          frame 4 {
          }
          frame 5 {
          }
          frame 6 {
          }
          frame 7 {
          }
          frame 8 {
          }
          frame 9 {
          }
          frame 10 {
          }
          frame 11 {
          }
          frame 12 {
          }
          frame 0, Default {
          }
        }
        n392 = case shown="4" w743 {
          tunnel: ["Full Vertical Binning" "Multi-Track" "Random-Track" "Single-Track" "Image"] -> w742
          frame 0, Default {
          }
          frame 1 {
          }
          frame 2 {
          }
          frame 3 {
          }
          frame 4 {
          }
        }
        n393 = case shown="2" w735 {
          tunnel: ["Fully Auto" "Open" "Closed"] -> w734
          frame 0, Default {
          }
          frame 1 {
          }
          frame 2 {
          }
        }
        n394 = case shown="1" w733 {
          tunnel: ["TTL Low" "TTL High"] -> w732
          frame 0, Default {
          }
          frame 1 {
          }
        }
        n395 = local read "Exposure time"() -> (w745:dbl)
        n396 = case shown="0, Default" w739 {
          tunnel: ["0.6" "2.2" "3.6" "4.33"] -> w738
          frame 0, Default {
          }
          frame 1 {
          }
          frame 2 {
          }
          frame 3 {
          }
        }
        n397 = case shown="2" w737 {
          tunnel: ["1" "2" "4"] -> w736
          frame 0, Default {
          }
          frame 1 {
          }
          frame 2 {
          }
        }
        n398 = Number To Fractional String(number=w745) -> (F-format string=w744:string)  [unwired: 3 in]
        n399 = local read "Cooler ON/OFF"() -> (w726:u16)
        n400 = local read "Time to open (ms)"() -> (w728:u16)
        n401 = local read "Time to close (ms)"() -> (w727:u16)
        n402 = local read "Horizontal binning"() -> (w715:u16)
        n403 = local read "Vertical binning"() -> (w716:u16)
        n404 = Bundle By Name(cluster=T16 {"Read Mode"="", "Acquisition Mode"="", "Trigger"="", "Exposure Time"="", "VShift Speed"="", "Readout rate"="", "Pre amp"="", "Shutter Mode"="", "Shutter TTL"="", "Time to open shutter"="", "Time to close shutter"="", "Cooler"="", "Temperature"="", "Initial Line"="", "Initial Column"="", "Final Line"="", "Final Column"="", "Horizontal binning"="", "Vertical binning"="", "Sub image"=""} ("Setup"), "Acquisition Mode"=w748, "Trigger"=w746, "Read Mode"=w742, "Exposure Time"=w744, "VShift Speed"=w738, "Readout rate"=w740, "Pre amp"=w736, "Shutter Mode"=w734, "Shutter TTL"=w732) -> (w731:T16)
        n405 = local read "Set temperature"() -> (w720:i8)
        n406 = local read "Initial Column"() -> (w718:u16)
        n407 = local read "Final Column"() -> (w714:u16)
        n408 = local read "Sub Image"() -> (w699:T3)
        n409 = local read "Final Line"() -> (w717:u16)
        n410 = local read "Initial Line"() -> (w719:u16)
        n411 = case shown="1" w726 {
          tunnel: ["OFF" "ON"] -> w725
          frame 0, Default {
          }
          frame 1 {
          }
        }
        n412 = case shown="\"64 x 64\"" w699 {
          tunnel: ["256 x 256" "512 x 512" "1024 x 1024" "Custom" "128 x 128" "64 x 64"] -> w698
          frame "256 x 256", Default {
          }
          frame "512 x 512" {
          }
          frame "1024 x 1024" {
          }
          frame "Custom" {
          }
          frame "128 x 128" {
          }
          frame "64 x 64" {
          }
        }
        n413 = Number To Decimal String(number=w728) -> (decimal integer string=w730:string)  [unwired: 1 in]
        n414 = Number To Decimal String(number=w727) -> (decimal integer string=w729:string)  [unwired: 1 in]
        n415 = Number To Decimal String(number=w720) -> (decimal integer string=w724:string)  [unwired: 1 in]
        n416 = Number To Decimal String(number=w719) -> (decimal integer string=w723:string)  [unwired: 1 in]
        n417 = Number To Decimal String(number=w718) -> (decimal integer string=w722:string)  [unwired: 1 in]
        n418 = Number To Decimal String(number=w717) -> (decimal integer string=w721:string)  [unwired: 1 in]
        n419 = Number To Decimal String(number=w714) -> (decimal integer string=w704:string)  [unwired: 1 in]
        n420 = Number To Decimal String(number=w715) -> (decimal integer string=w703:string)  [unwired: 1 in]
        n421 = Number To Decimal String(number=w716) -> (decimal integer string=w702:string)  [unwired: 1 in]
        n422 = Bundle By Name(cluster=w731, "Time to open shutter"=w730, "Time to close shutter"=w729, "Cooler"=w725, "Temperature"=w724, "Initial Line"=w723, "Initial Column"=w722, "Final Line"=w721, "Final Column"=w704, "Horizontal binning"=w703, "Vertical binning"=w702, "Sub image"=w698) -> (w700:T16)
        n423 = call "Write File Setup.vi"("error in (no error)"=w712, "Setup"=w700, "Setup File in"=w713) -> ("error out"=w711:errorcluster, "Setup File out"=w710:refnum<class "Setup File.lvclass">)  [unwired: 7 in]
        n424 = call "Write File.vi"("error in (no error)"=w711, "Setup File in"=w710) -> ("error out"=w708:errorcluster, "Setup File out"=w709:refnum<class "Setup File.lvclass">)  [unwired: 8 in]
        n425 = call "Write Setup File.lvclass.vi"("error in (no error)"=w708, "Setup File.lvclass"=w709, "Application in"=w707) -> ("error out"=w706:errorcluster, "Application out"=w705:refnum<class "Application.lvclass">)  [unwired: 7 in]
      }
      event "Sub Image": Value Change {
        w810 = cluster{dbl, dbl} {0.0, 0.0}
        # "Esta operação escreve a configuração do binning da imagem na janela gráfica binning de acordo com as opções pré-programadas pelo indicador Sub Image."
        n426 = event-data() -> ()  [unwired: 1 in, 1 out]
        n427 = case shown="\"128 x 128\"" "Sub Image" {
          tunnel: [128 256 512 512 64 32] -> w804
          frame "256 x 256", Default {
            w829 = 128
            n428 = property on="Binning" class="XYGraph (strict)"() -> ("XScale.Maximum"=w834:dbl)  [unwired: 2 in, 2 out]
            n429 = property on="Binning" class="XYGraph (strict)"() -> ("YScale.Maximum"=w833:dbl)  [unwired: 2 in, 2 out]
            n430 = Divide(x=w834, y=2) -> (x/y=w831:dbl)
            n431 = Divide(x=w833, y=2) -> (x/y=w830:dbl)
            n432 = Add(x=w831, y=w829) -> (x+y=w827:dbl)
            n433 = Subtract(x=w831, y=w829) -> (x-y=w824:dbl)
            n434 = Subtract(x=w830, y=w829) -> (x-y=w823:dbl)
            n435 = Add(x=w830, y=w829) -> (x+y=w828:dbl)
            n436 = Increment(x=w823) -> (x+1=w826:dbl)
            n437 = Increment(x=w824) -> (x+1=w825:dbl)
            n438 = property on="Initial Line" class="DigNum (strict)"("DisabledEnum"=T17."Disabled and Grayed Out" ("Disabled")) -> ()  [unwired: 2 in, 2 out]
            n439 = property on="Initial Column" class="DigNum (strict)"("DisabledEnum"=T17."Disabled and Grayed Out" ("Disabled")) -> ()  [unwired: 2 in, 2 out]
            n440 = property on="Final Line" class="DigNum (strict)"("DisabledEnum"=T17."Disabled and Grayed Out" ("Disabled")) -> ()  [unwired: 2 in, 2 out]
            n441 = property on="Final Column" class="DigNum (strict)"("DisabledEnum"=T17."Disabled and Grayed Out" ("Disabled")) -> ()  [unwired: 2 in, 2 out]
            n442 = local write "Final Line"(w827) -> ()
            n443 = local write "Initial Line"(w825) -> ()
            n444 = local write "Initial Column"(w826) -> ()
            n445 = local write "Final Column"(w828) -> ()
          }
          frame "512 x 512" {
            w847 = 256
            n446 = property on="Binning" class="XYGraph (strict)"() -> ("XScale.Maximum"=w852:dbl)  [unwired: 2 in, 2 out]
            n447 = property on="Binning" class="XYGraph (strict)"() -> ("YScale.Maximum"=w851:dbl)  [unwired: 2 in, 2 out]
            n448 = Divide(x=w852, y=2) -> (x/y=w849:dbl)
            n449 = Divide(x=w851, y=2) -> (x/y=w848:dbl)
            n450 = Add(x=w849, y=w847) -> (x+y=w845:dbl)
            n451 = Subtract(x=w849, y=w847) -> (x-y=w842:dbl)
            n452 = Subtract(x=w848, y=w847) -> (x-y=w841:dbl)
            n453 = Add(x=w848, y=w847) -> (x+y=w846:dbl)
            n454 = Increment(x=w841) -> (x+1=w844:dbl)
            n455 = Increment(x=w842) -> (x+1=w843:dbl)
            n456 = property on="Initial Line" class="DigNum (strict)"("DisabledEnum"=T17."Disabled and Grayed Out" ("Disabled")) -> ()  [unwired: 2 in, 2 out]
            n457 = property on="Initial Column" class="DigNum (strict)"("DisabledEnum"=T17."Disabled and Grayed Out" ("Disabled")) -> ()  [unwired: 2 in, 2 out]
            n458 = property on="Final Line" class="DigNum (strict)"("DisabledEnum"=T17."Disabled and Grayed Out" ("Disabled")) -> ()  [unwired: 2 in, 2 out]
            n459 = property on="Final Column" class="DigNum (strict)"("DisabledEnum"=T17."Disabled and Grayed Out" ("Disabled")) -> ()  [unwired: 2 in, 2 out]
            n460 = local write "Final Line"(w845) -> ()
            n461 = local write "Initial Line"(w843) -> ()
            n462 = local write "Initial Column"(w844) -> ()
            n463 = local write "Final Column"(w846) -> ()
          }
          frame "1024 x 1024" {
            w865 = 512
            n464 = property on="Binning" class="XYGraph (strict)"() -> ("XScale.Maximum"=w870:dbl)  [unwired: 2 in, 2 out]
            n465 = property on="Binning" class="XYGraph (strict)"() -> ("YScale.Maximum"=w869:dbl)  [unwired: 2 in, 2 out]
            n466 = Divide(x=w870, y=2) -> (x/y=w867:dbl)
            n467 = Divide(x=w869, y=2) -> (x/y=w866:dbl)
            n468 = Add(x=w867, y=w865) -> (x+y=w863:dbl)
            n469 = Subtract(x=w867, y=w865) -> (x-y=w860:dbl)
            n470 = Subtract(x=w866, y=w865) -> (x-y=w859:dbl)
            n471 = Add(x=w866, y=w865) -> (x+y=w864:dbl)
            n472 = Increment(x=w859) -> (x+1=w862:dbl)
            n473 = Increment(x=w860) -> (x+1=w861:dbl)
            n474 = property on="Initial Line" class="DigNum (strict)"("DisabledEnum"=T17."Disabled and Grayed Out" ("Disabled")) -> ()  [unwired: 2 in, 2 out]
            n475 = property on="Initial Column" class="DigNum (strict)"("DisabledEnum"=T17."Disabled and Grayed Out" ("Disabled")) -> ()  [unwired: 2 in, 2 out]
            n476 = property on="Final Line" class="DigNum (strict)"("DisabledEnum"=T17."Disabled and Grayed Out" ("Disabled")) -> ()  [unwired: 2 in, 2 out]
            n477 = property on="Final Column" class="DigNum (strict)"("DisabledEnum"=T17."Disabled and Grayed Out" ("Disabled")) -> ()  [unwired: 2 in, 2 out]
            n478 = local write "Final Line"(w863) -> ()
            n479 = local write "Initial Line"(w861) -> ()
            n480 = local write "Initial Column"(w862) -> ()
            n481 = local write "Final Column"(w864) -> ()
          }
          frame "Custom" {
            w879 = 1
            n482 = call <userlib>:"GetDetector.vi"() -> ("ypixels"=w877:i32, "xpixels"=w878:i32)  [unwired: 4 in, 2 out]
            n483 = property on="Initial Line" class="DigNum (strict)"("DisabledEnum"=T17."Enabled" ("Disabled")) -> ()  [unwired: 2 in, 2 out]
            n484 = property on="Initial Column" class="DigNum (strict)"("DisabledEnum"=T17."Enabled" ("Disabled")) -> ()  [unwired: 2 in, 2 out]
            n485 = property on="Final Line" class="DigNum (strict)"("DisabledEnum"=T17."Enabled" ("Disabled")) -> ()  [unwired: 2 in, 2 out]
            n486 = property on="Final Column" class="DigNum (strict)"("DisabledEnum"=T17."Enabled" ("Disabled")) -> ()  [unwired: 2 in, 2 out]
            n487 = local write "Final Line"(w878) -> ()
            n488 = local write "Initial Line"(w879) -> ()
            n489 = local write "Initial Column"(w879) -> ()
            n490 = local write "Final Column"(w877) -> ()
          }
          frame "128 x 128" {
            w891 = 64
            n491 = property on="Binning" class="XYGraph (strict)"() -> ("XScale.Maximum"=w896:dbl)  [unwired: 2 in, 2 out]
            n492 = property on="Binning" class="XYGraph (strict)"() -> ("YScale.Maximum"=w895:dbl)  [unwired: 2 in, 2 out]
            n493 = Divide(x=w896, y=2) -> (x/y=w893:dbl)
            n494 = Divide(x=w895, y=2) -> (x/y=w892:dbl)
            n495 = Add(x=w893, y=w891) -> (x+y=w889:dbl)
            n496 = Subtract(x=w893, y=w891) -> (x-y=w886:dbl)
            n497 = Subtract(x=w892, y=w891) -> (x-y=w888:dbl)
            n498 = Add(x=w892, y=w891) -> (x+y=w890:dbl)
            n499 = Increment(x=w888) -> (x+1=w887:dbl)
            n500 = Increment(x=w886) -> (x+1=w885:dbl)
            n501 = property on="Initial Line" class="DigNum (strict)"("DisabledEnum"=T17."Disabled and Grayed Out" ("Disabled")) -> ()  [unwired: 2 in, 2 out]
            n502 = property on="Initial Column" class="DigNum (strict)"("DisabledEnum"=T17."Disabled and Grayed Out" ("Disabled")) -> ()  [unwired: 2 in, 2 out]
            n503 = property on="Final Line" class="DigNum (strict)"("DisabledEnum"=T17."Disabled and Grayed Out" ("Disabled")) -> ()  [unwired: 2 in, 2 out]
            n504 = property on="Final Column" class="DigNum (strict)"("DisabledEnum"=T17."Disabled and Grayed Out" ("Disabled")) -> ()  [unwired: 2 in, 2 out]
            n505 = local write "Final Line"(w889) -> ()
            n506 = local write "Initial Line"(w885) -> ()
            n507 = local write "Initial Column"(w887) -> ()
            n508 = local write "Final Column"(w890) -> ()
          }
          frame "64 x 64" {
            w909 = 32
            n509 = property on="Binning" class="XYGraph (strict)"() -> ("XScale.Maximum"=w914:dbl)  [unwired: 2 in, 2 out]
            n510 = property on="Binning" class="XYGraph (strict)"() -> ("YScale.Maximum"=w913:dbl)  [unwired: 2 in, 2 out]
            n511 = Divide(x=w914, y=2) -> (x/y=w911:dbl)
            n512 = Divide(x=w913, y=2) -> (x/y=w910:dbl)
            n513 = Add(x=w911, y=w909) -> (x+y=w907:dbl)
            n514 = Subtract(x=w911, y=w909) -> (x-y=w904:dbl)
            n515 = Subtract(x=w910, y=w909) -> (x-y=w903:dbl)
            n516 = Add(x=w910, y=w909) -> (x+y=w908:dbl)
            n517 = Increment(x=w903) -> (x+1=w906:dbl)
            n518 = Increment(x=w904) -> (x+1=w905:dbl)
            n519 = property on="Initial Line" class="DigNum (strict)"("DisabledEnum"=T17."Disabled and Grayed Out" ("Disabled")) -> ()  [unwired: 2 in, 2 out]
            n520 = property on="Initial Column" class="DigNum (strict)"("DisabledEnum"=T17."Disabled and Grayed Out" ("Disabled")) -> ()  [unwired: 2 in, 2 out]
            n521 = property on="Final Line" class="DigNum (strict)"("DisabledEnum"=T17."Disabled and Grayed Out" ("Disabled")) -> ()  [unwired: 2 in, 2 out]
            n522 = property on="Final Column" class="DigNum (strict)"("DisabledEnum"=T17."Disabled and Grayed Out" ("Disabled")) -> ()  [unwired: 2 in, 2 out]
            n523 = local write "Final Line"(w907) -> ()
            n524 = local write "Initial Line"(w905) -> ()
            n525 = local write "Initial Column"(w906) -> ()
            n526 = local write "Final Column"(w908) -> ()
          }
        }
        n527 = property on="Binning" class="XYGraph (strict)"() -> ("XScale.Maximum"=w808:dbl)  [unwired: 2 in, 2 out]
        n528 = property on="Binning" class="XYGraph (strict)"() -> ("YScale.Maximum"=w806:dbl)  [unwired: 2 in, 2 out]
        n529 = Divide(x=w806, y=2) -> (x/y=w814:dbl)
        n530 = Divide(x=w808, y=2) -> (x/y=w815:dbl)
        n531 = Subtract(x=w815, y=w804) -> (x-y=w812:dbl)
        n532 = Add(x=w804, y=w815) -> (x+y=w813:dbl)
        n533 = Add(x=w804, y=w814) -> (x+y=w811:dbl)
        n534 = Subtract(x=w814, y=w804) -> (x-y=w809:dbl)
        n535 = Bundle(cluster=w810, w812, w809) -> (w822:cluster{dbl, dbl})
        n536 = Bundle(cluster=w810, w813, w809) -> (w821:cluster{dbl, dbl})
        n537 = Bundle(cluster=w810, w813, w811) -> (w820:cluster{dbl, dbl})
        n538 = Bundle(cluster=w810, w812, w811) -> (w819:cluster{dbl, dbl})
        n539 = Bundle(cluster=w810, w809, w809) -> (w818:cluster{dbl, dbl})
        n540 = Build Array(w822, w821, w820, w819, w818) -> (→"Binning":cluster{dbl, dbl}[])
      }
      event "FITS": Value Change {
        n541 = event-data() -> ()  [unwired: 1 in, 2 out]
        n542 = case shown="True" "FITS" {
          tunnel: [_ "FITS"] -> w923
          frame False {
          }
          frame True {
            w929 = FALSE ("SIF")
            n543 = local write "SIF"(w929) -> ()
            n544 = local write "TIFF"(w929) -> ()
            n545 = property on="FITS Format" class="Ring (strict)"("DisabledEnum"=T17."Enabled" ("Disabled")) -> ()  [unwired: 2 in, 2 out]
            n546 = property on="Tiff Position" class="DigNum (strict)"("DisabledEnum"=T17."Disabled and Grayed Out" ("Disabled")) -> ()  [unwired: 2 in, 2 out]
            n547 = property on="Tiff Type" class="Ring (strict)"("DisabledEnum"=T17."Disabled and Grayed Out" ("Disabled")) -> ()  [unwired: 2 in, 2 out]
          }
        }
        n548 = local write "Image Format"(w923) -> ()
      }
      event "SIF": Value Change {
        n549 = event-data() -> ()  [unwired: 1 in, 2 out]
        n550 = case shown="True" "SIF" {
          tunnel: [_ "SIF"] -> w932
          frame False {
          }
          frame True {
            w938 = FALSE ("SIF")
            n551 = local write "FITS"(w938) -> ()
            n552 = local write "TIFF"(w938) -> ()
            n553 = property on="Tiff Position" class="DigNum (strict)"("DisabledEnum"=T17."Disabled and Grayed Out" ("Disabled")) -> ()  [unwired: 2 in, 2 out]
            n554 = property on="Tiff Type" class="Ring (strict)"("DisabledEnum"=T17."Disabled and Grayed Out" ("Disabled")) -> ()  [unwired: 2 in, 2 out]
            n555 = property on="FITS Format" class="Ring (strict)"("DisabledEnum"=T17."Disabled and Grayed Out" ("Disabled")) -> ()  [unwired: 2 in, 2 out]
          }
        }
        n556 = local write "Image Format"(w932) -> ()
      }
      event "TIFF": Value Change {
        n557 = event-data() -> ()  [unwired: 1 in, 2 out]
        n558 = case shown="True" "TIFF" {
          tunnel: [_ "TIFF"] -> w941
          frame False {
          }
          frame True {
            w947 = FALSE ("SIF")
            n559 = local write "FITS"(w947) -> ()
            n560 = local write "SIF"(w947) -> ()
            n561 = property on="Tiff Position" class="DigNum (strict)"("DisabledEnum"=T17."Enabled" ("Disabled")) -> ()  [unwired: 2 in, 2 out]
            n562 = property on="Tiff Type" class="Ring (strict)"("DisabledEnum"=T17."Enabled" ("Disabled")) -> ()  [unwired: 2 in, 2 out]
            n563 = property on="FITS Format" class="Ring (strict)"("DisabledEnum"=T17."Disabled and Grayed Out" ("Disabled")) -> ()  [unwired: 2 in, 2 out]
          }
        }
        n564 = local write "Image Format"(w941) -> ()
      }
      event "Initial Line", "Initial Column", "Final Line", "Final Column": Value Change {
        w955 = cluster{dbl, dbl} {0.0, 0.0}
        # "Esta operação escreve na janela gráfica do Binning da imagem a configuração escolhida pelo usuário."
        n565 = event-data() -> ()  [unwired: 1 in, 2 out]
        n566 = local read "Initial Column"() -> (w951:u16)
        n567 = local read "Final Column"() -> (w954:u16)
        n568 = local read "Initial Line"() -> (w952:u16)
        n569 = local read "Final Line"() -> (w953:u16)
        n570 = Bundle(cluster=w955, w952, w951) -> (w960:cluster{dbl, dbl})
        n571 = Bundle(cluster=w955, w952, w954) -> (w959:cluster{dbl, dbl})
        n572 = Bundle(cluster=w955, w953, w954) -> (w958:cluster{dbl, dbl})
        n573 = Bundle(cluster=w955, w953, w951) -> (w957:cluster{dbl, dbl})
        n574 = Bundle(cluster=w955, w952, w951) -> (w956:cluster{dbl, dbl})
        n575 = Build Array(w960, w959, w958, w957, w956) -> (w950:cluster{dbl, dbl}[])
        n576 = local write "Binning"(w950) -> ()
      }
      event "Sync Mode": Value Change {
        # "Esta operação apresenta uma interface para a escolha do modo de sincronização das câmeras quando o botão Sync Mode for pressionado."
        n577 = event-data() -> ()  [unwired: 1 in, 1 out]
        n578 = call "Write Sync Mode.vi"("error in (no error)"=w964, "Application in"=w963) -> ("error out"=w962:errorcluster, "Application out"=w961:refnum<class "Application.lvclass">)  [unwired: 8 in]
      }
      event "Set temperature": Value Change {
        # "Quando a temperatura do CCD for alterada, esta operação enviará a informação da nova temperatura para o controlador da câmera."
        n579 = event-data() -> ()  [unwired: 1 in, 1 out]
        n580 = call "Read RxTxCamera.lvclass.vi"("error in (no error)"=w983, "Application in"=w982) -> ("error out"=w981:errorcluster, "RxTxCamera.lvclass"=w980:refnum<class "RxTxCamera.lvclass">, "Application out"=w968:refnum<class "Application.lvclass">)  [unwired: 7 in]
        n581 = Bundle By Name(cluster=T7 {"Cooler ON/OFF"=0, "Set temperature"=20.0, "Shutter Mode "=2, "Shutter TTL"=0, "Time to open (ms)"=50.0, "Time to close (ms)"=50.0, "Pre-amplifier gain"=0, "Vertical clock\n  voltage amplitude"=0, "Vertical Shift Speed"=3, "Readout Rate "=1, "Trigger "=0, "Conventional/EM"=1, "Read Mode "=4, "Acquisition Mode "=1, "Exposure Time (s) "=0.0, "Initial Line"=1, "Initial Column"=1, "Final Line"=1024, "Final Column"=1024, "Horizontal binning"=1, "Vertical binning "=1, "FITS Format"=0, "Image Format"="FITS", "Tiff Position "=1, "Tiff Type"=0, "Image Path"=""} ("RED Channel Settings"), "Set temperature"="Set temperature") -> (w979:T7)
        n582 = call "Write Config String.vi"("error in (no error)"=w981, "RED Channel Settings"=w979, "RxTxCamera in"=w980) -> ("error out"=w977:errorcluster, "RxTxCamera out"=w976:refnum<class "RxTxCamera.lvclass">)  [unwired: 7 in]
        n583 = call "Enqeue message.vi"("error in (no error)"=w977, "RxTx in"=w976) -> ("error out"=w974:errorcluster, "RxTx out"=w973:refnum<class "RxTxCamera.lvclass">)  [unwired: 8 in]
        n584 = call "Write Command String.vi"("error in (no error)"=w974, "Command String"="SET TEMP", "RxTxCamera in"=w973) -> ("error out"=w972:errorcluster, "RxTxCamera out"=w971:refnum<class "RxTxCamera.lvclass">)  [unwired: 7 in]
        n585 = call "Enqeue message.vi"("error in (no error)"=w972, "RxTx in"=w971) -> ("error out"=w970:errorcluster, "RxTx out"=w969:refnum<class "RxTxCamera.lvclass">)  [unwired: 8 in]
        n586 = call "Write RxTxCamera.lvclass.vi"("error in (no error)"=w970, "RxTxCamera.lvclass"=w969, "Application in"=w968) -> ("error out"=w967:errorcluster, "Application out"=w966:refnum<class "Application.lvclass">)  [unwired: 7 in]
        "Temperature ºC" <- "Set temperature"
      }
      event "Exposure time": Value Change {
        n587 = event-data() -> ()  [unwired: 1 in, 1 out]
        n588 = local read "Exposure time"() -> (w986:dbl)
        n589 = local write "Exposure Time (s)  2"(w986) -> ()
      }
      event "Exposure Time (s)  2": Value Change {
        n590 = event-data() -> ()  [unwired: 1 in, 1 out]
        n591 = local write "Exposure time"("Exposure Time (s)  2") -> ()
      }
      event "Cooler ON/OFF": Value Change {
        # "Esta operação é responsável por enviar uma mensagem para o controlador da câmera Ligar/Desligar o cooler"
        n592 = event-data() -> ()  [unwired: 1 in, 1 out]
        n593 = call "Read RxTxCamera.lvclass.vi"("error in (no error)"=w997, "Application in"=w996) -> ("error out"=w1000:errorcluster, "RxTxCamera.lvclass"=w999:refnum<class "RxTxCamera.lvclass">, "Application out"=w998:refnum<class "Application.lvclass">)  [unwired: 7 in]
        n594 = case shown="0, Default" "Cooler ON/OFF" {
          selector: "Cooler ON/OFF" -> [w1005 w1020]
          tunnel: w1000 -> [w1007 w1030]
          tunnel: w999 -> [w1006 w1029]
          tunnel: w998 -> [w1004 w1018]
          tunnel: [w1004 w1018] -> w994
          tunnel: [w1003 w1017] -> w992
          tunnel: [w1002 w1019] -> w993
          frame 0, Default {
            n595 = Bundle By Name(cluster=T7 {"Cooler ON/OFF"=0, "Set temperature"=20.0, "Shutter Mode "=2, "Shutter TTL"=0, "Time to open (ms)"=50.0, "Time to close (ms)"=50.0, "Pre-amplifier gain"=0, "Vertical clock\n  voltage amplitude"=0, "Vertical Shift Speed"=3, "Readout Rate "=1, "Trigger "=0, "Conventional/EM"=1, "Read Mode "=4, "Acquisition Mode "=1, "Exposure Time (s) "=0.0, "Initial Line"=1, "Initial Column"=1, "Final Line"=1024, "Final Column"=1024, "Horizontal binning"=1, "Vertical binning "=1, "FITS Format"=0, "Image Format"="FITS", "Tiff Position "=1, "Tiff Type"=0, "Image Path"=""} ("RED Channel Settings"), "Cooler ON/OFF"=w1005) -> (w1015:T7)
            n596 = call "Write Config String.vi"("error in (no error)"=w1007, "RED Channel Settings"=w1015, "RxTxCamera in"=w1006) -> ("error out"=w1014:errorcluster, "RxTxCamera out"=w1013:refnum<class "RxTxCamera.lvclass">)  [unwired: 7 in]
            n597 = call "Enqeue message.vi"("error in (no error)"=w1014, "RxTx in"=w1013) -> ("error out"=w1011:errorcluster, "RxTx out"=w1010:refnum<class "RxTxCamera.lvclass">)  [unwired: 8 in]
            n598 = call "Write Command String.vi"("error in (no error)"=w1011, "Command String"="TURN COOLER OFF", "RxTxCamera in"=w1010) -> ("error out"=w1009:errorcluster, "RxTxCamera out"=w1008:refnum<class "RxTxCamera.lvclass">)  [unwired: 7 in]
            n599 = call "Enqeue message.vi"("error in (no error)"=w1009, "RxTx in"=w1008) -> ("error out"=w1003:errorcluster, "RxTx out"=w1002:refnum<class "RxTxCamera.lvclass">)  [unwired: 8 in]
          }
          frame 1 {
            n600 = Bundle By Name(cluster=T7 {"Cooler ON/OFF"=0, "Set temperature"=20.0, "Shutter Mode "=2, "Shutter TTL"=0, "Time to open (ms)"=50.0, "Time to close (ms)"=50.0, "Pre-amplifier gain"=0, "Vertical clock\n  voltage amplitude"=0, "Vertical Shift Speed"=3, "Readout Rate "=1, "Trigger "=0, "Conventional/EM"=1, "Read Mode "=4, "Acquisition Mode "=1, "Exposure Time (s) "=0.0, "Initial Line"=1, "Initial Column"=1, "Final Line"=1024, "Final Column"=1024, "Horizontal binning"=1, "Vertical binning "=1, "FITS Format"=0, "Image Format"="FITS", "Tiff Position "=1, "Tiff Type"=0, "Image Path"=""} ("RED Channel Settings"), "Cooler ON/OFF"=w1020) -> (w1028:T7)
            n601 = call "Write Config String.vi"("error in (no error)"=w1030, "RED Channel Settings"=w1028, "RxTxCamera in"=w1029) -> ("error out"=w1027:errorcluster, "RxTxCamera out"=w1026:refnum<class "RxTxCamera.lvclass">)  [unwired: 7 in]
            n602 = call "Enqeue message.vi"("error in (no error)"=w1027, "RxTx in"=w1026) -> ("error out"=w1024:errorcluster, "RxTx out"=w1023:refnum<class "RxTxCamera.lvclass">)  [unwired: 8 in]
            n603 = call "Write Command String.vi"("error in (no error)"=w1024, "Command String"="TURN COOLER ON", "RxTxCamera in"=w1023) -> ("error out"=w1022:errorcluster, "RxTxCamera out"=w1021:refnum<class "RxTxCamera.lvclass">)  [unwired: 7 in]
            n604 = call "Enqeue message.vi"("error in (no error)"=w1022, "RxTx in"=w1021) -> ("error out"=w1017:errorcluster, "RxTx out"=w1019:refnum<class "RxTxCamera.lvclass">)  [unwired: 8 in]
          }
        }
        n605 = call "Write RxTxCamera.lvclass.vi"("error in (no error)"=w992, "RxTxCamera.lvclass"=w993, "Application in"=w994) -> ("error out"=w990:errorcluster, "Application out"=w991:refnum<class "Application.lvclass">)  [unwired: 7 in]
      }
      event "BIAS": Value Change {
        w1038 = FALSE
        # "Quando o botão BIAS é pressionado, esta operação fará a leitura do arquivo Bias.txt e escreverá o conteúdo do arquivo na interface."
        n606 = event-data() -> ()  [unwired: 1 in, 1 out]
        n607 = local write "COMP"(w1038) -> ()
        n608 = local write "FLAT"(w1038) -> ()
        n609 = case shown="True" "BIAS" {
          tunnel: [_ "BIAS"] -> w1031
          tunnel: w1035 -> [w1041 w1057]
          tunnel: w1034 -> [w1040 w1056]
          tunnel: [w1041 w1050] -> w1033
          tunnel: [w1040 w1051] -> w1032
          frame False {
          }
          frame True {
            n610 = call "Read Setup File.lvclass.vi"("error in (no error)"=w1057, "Application in"=w1056) -> ("error out"=w1049:errorcluster, "Setup File.lvclass"=w1048:refnum<class "Setup File.lvclass">, "Application out"=w1052:refnum<class "Application.lvclass">)  [unwired: 7 in]
            n611 = call "Write File Name.vi"("error in (no error)"=w1049, "File Name"="Bias.txt", "Setup File in"=w1048) -> ("error out"=w1054:errorcluster, "Setup File out"=w1053:refnum<class "Setup File.lvclass">)  [unwired: 7 in]
            n612 = call "Read File.vi"("error in (no error)"=w1054, "Setup File in"=w1053) -> ("error out"=w1046:errorcluster, "Setup"=w1047:T16, "Setup File out"=w1043:refnum<class "Setup File.lvclass">)  [unwired: 7 in]
            n613 = call "Read File Path.vi"("error in (no error)"=w1046, "Setup File in"=w1043) -> ("error out"=w1045:errorcluster, "File Path"=w1042:string, "Setup File out"=w1044:refnum<class "Setup File.lvclass">)  [unwired: 7 in]
            n614 = local write "Setup File Path:"(w1042) -> ()
            n615 = stacked-sequence {
              tunnel: w1047 -> [w1063 w1076 w1088 w1099 w1112]
              frame #0 {
                n616 = Unbundle By Name(w1063) -> ("Read Mode"=w1060:string)
                n617 = To Upper Case(1:w1060) -> (0:w1064:string)
                n618 = Concatenate Strings("Invalid Read Mode value: ", w1060) -> (w1059:string)
                n619 = case shown="\"False\", Default" w1064 {
                  tunnel: [_ _ w1067 w1068 w1069 w1070 w1071] -> w1062
                  tunnel: w1059 -> [w1065 _ _ _ _ _ _]
                  frame "False", Default {
                    n620 = One Button Dialog(message=w1065, button name ("OK")="OK") -> ()  [unwired: 1 out]
                  }
                  frame "" {
                  }
                  frame "FULLVERTICALBINNING " {
                    w1067 = u16 0 items=["Full Vertical Binning", "Multi-Track", "Random-Track", "Single-Track", "Image"] ("Read Mode")
                  }
                  frame "MULTI-TRACK" {
                    w1068 = u16 1 items=["Full Vertical Binning", "Multi-Track", "Random-Track", "Single-Track", "Image"] ("Read Mode")
                  }
                  frame "RANDOM-TRACK" {
                    w1069 = u16 2 items=["Full Vertical Binning", "Multi-Track", "Random-Track", "Single-Track", "Image"] ("Read Mode")
                  }
                  frame "SINGLE-TRACK" {
                    w1070 = u16 3 items=["Full Vertical Binning", "Multi-Track", "Random-Track", "Single-Track", "Image"] ("Read Mode")
                  }
                  frame "IMAGE" {
                    w1071 = u16 4 items=["Full Vertical Binning", "Multi-Track", "Random-Track", "Single-Track", "Image"] ("Read Mode")
                  }
                }
                n621 = local write "Read Mode"(w1062) -> ()
              }
              frame #1 {
                n622 = Unbundle By Name(w1076) -> ("Exposure Time"=w1077:string)
                n623 = Fract/Exp String To Number(string=w1077) -> (number=w1073:dbl)  [unwired: 3 in, 1 out]
                n624 = Less?(x=w1073, y=0.0) -> (x < y?=w1074:bool)
                n625 = case shown="True" w1074 {
                  tunnel: w1073 -> [w1078 w1081]
                  tunnel: "Exposure time lower than zero: " -> [_ w1079]
                  frame False {
                    n626 = local write "Exposure time"(w1078) -> ()
                    n627 = local write "Exposure Time (s)  2"(w1078) -> ()
                  }
                  frame True {
                    n628 = Number To Fractional String(number=w1081) -> (F-format string=w1080:string)  [unwired: 3 in]
                    n629 = Concatenate Strings(w1079, w1080) -> (w1082:string)
                    n630 = One Button Dialog(message=w1082, button name ("OK")="OK") -> ()  [unwired: 1 out]
                  }
                }
              }
              frame #2 {
                n631 = Unbundle By Name(w1088) -> ("Shutter Mode"=w1086:string)
                n632 = Concatenate Strings("Invalid Shutter Mode value: ", w1086) -> (w1084:string)
                n633 = To Upper Case(1:w1086) -> (0:w1089:string)
                n634 = case shown="\"False\", Default" w1089 {
                  tunnel: [_ _ w1092 w1093 w1094] -> w1087
                  tunnel: w1084 -> [w1090 _ _ _ _]
                  frame "False", Default {
                    n635 = One Button Dialog(message=w1090, button name ("OK")="OK") -> ()  [unwired: 1 out]
                  }
                  frame "" {
                  }
                  frame "FULLYAUTO" {
                    w1092 = u16 0 items=["Fully Auto", "OPEN", "CLOSED"] ("Shutter Mode")
                  }
                  frame "OPEN" {
                    w1093 = u16 1 items=["Fully Auto", "OPEN", "CLOSED"] ("Shutter Mode")
                  }
                  frame "CLOSED" {
                    w1094 = u16 2 items=["Fully Auto", "OPEN", "CLOSED"] ("Shutter Mode")
                  }
                }
                n636 = local write "Shutter Mode"(w1087) -> ()
              }
              frame #3 {
                n637 = Unbundle By Name(w1099) -> ("Shutter TTL"=w1096:string)
                n638 = To Upper Case(1:w1096) -> (0:w1100:string)
                n639 = Concatenate Strings("Invalid Shutter TTL value: ", w1096) -> (w1095:string)
                n640 = case shown="\"TTLHIGH\"" w1100 {
                  tunnel: [_ _ w1103 w1104] -> w1098
                  tunnel: w1095 -> [w1101 _ _ _]
                  frame "False", Default {
                    n641 = One Button Dialog(message=w1101, button name ("OK")="OK") -> ()  [unwired: 1 out]
                  }
                  frame "" {
                  }
                  frame "TTLHIGH" {
                    w1103 = u16 1 items=["TTL Low", "TTL High"] ("Shutter TTL")
                  }
                  frame "TTLLOW" {
                    w1104 = u16 0 items=["TTL Low", "TTL High"] ("Shutter TTL")
                  }
                }
                n642 = local write "Shutter TTL"(w1098) -> ()
              }
              frame #4 {
                n643 = Unbundle By Name(w1112) -> ("Time to open shutter"=w1113:string, "Time to close shutter"=w1111:string)
                n644 = Decimal String To Number(string=w1113) -> (number=w1107:i32)  [unwired: 2 in, 1 out]
                n645 = Decimal String To Number(string=w1111) -> (number=w1105:i32)  [unwired: 2 in, 1 out]
                n646 = Less?(x=w1107, y=50) -> (x < y?=w1108:bool)
                n647 = Less?(x=w1105, y=50) -> (x < y?=w1106:bool)
                n648 = case shown="True" w1108 {
                  tunnel: w1107 -> [w1120 w1121]
                  frame False {
                    n649 = local write "Time to open (ms)"(w1120) -> ()
                  }
                  frame True {
                    n650 = Number To Decimal String(number=w1121) -> (decimal integer string=w1122:string)  [unwired: 1 in]
                    n651 = Concatenate Strings("Time to open shutter is lower than 50 ms: ", w1122) -> (w1124:string)
                    n652 = One Button Dialog(message=w1124, button name ("OK")="OK") -> ()  [unwired: 1 out]
                  }
                }
                n653 = case shown="True" w1106 {
                  tunnel: w1105 -> [w1114 w1115]
                  frame False {
                    n654 = local write "Time to close (ms)"(w1114) -> ()
                  }
                  frame True {
                    n655 = Number To Decimal String(number=w1115) -> (decimal integer string=w1116:string)  [unwired: 1 in]
                    n656 = Concatenate Strings("Time to close shutter is lower than 50 ms: ", w1116) -> (w1118:string)
                    n657 = One Button Dialog(message=w1118, button name ("OK")="OK") -> ()  [unwired: 1 out]
                  }
                }
              }
            }
            n658 = call "Write Setup File.lvclass.vi"("error in (no error)"=w1045, "Setup File.lvclass"=w1044, "Application in"=w1052) -> ("error out"=w1050:errorcluster, "Application out"=w1051:refnum<class "Application.lvclass">)  [unwired: 7 in]
          }
        }
        n659 = call "Write Observation type.vi"("error in (no error)"=w1033, "Observation type"=w1031, "Application in"=w1032) -> ("error out"=w1037:errorcluster, "Application out"=w1036:refnum<class "Application.lvclass">)  [unwired: 7 in]
      }
      event "FLAT": Value Change {
        w1128 = FALSE
        n660 = event-data() -> ()  [unwired: 1 in, 1 out]
        n661 = case shown="True" "FLAT" {
          tunnel: [_ "FLAT"] -> w1129
          frame False {
          }
          frame True {
          }
        }
        n662 = local write "BIAS"(w1128) -> ()
        n663 = local write "COMP"(w1128) -> ()
        n664 = call "Write Observation type.vi"("error in (no error)"=w1131, "Observation type"=w1129, "Application in"=w1130) -> ("error out"=w1127:errorcluster, "Application out"=w1126:refnum<class "Application.lvclass">)  [unwired: 7 in]
      }
      event "COMP": Value Change {
        w1134 = FALSE
        n665 = event-data() -> ()  [unwired: 1 in, 1 out]
        n666 = case shown="True" "COMP" {
          tunnel: [_ "COMP"] -> w1137
          frame False {
          }
          frame True {
          }
        }
        n667 = local write "FLAT"(w1134) -> ()
        n668 = local write "BIAS"(w1134) -> ()
        n669 = call "Write Observation type.vi"("error in (no error)"=w1139, "Observation type"=w1137, "Application in"=w1138) -> ("error out"=w1136:errorcluster, "Application out"=w1135:refnum<class "Application.lvclass">)  [unwired: 7 in]
      }
      event "Stop Button": Value Change {
        # "Quando o botão stop é pressionado, a interface manda um comando para as câmeras desligarem."
        n670 = event-data() -> ()  [unwired: 1 in, 1 out]
        n671 = call "Read RxTxCamera.lvclass.vi"("Application in"=w1152) -> ("error out"=w1147:errorcluster, "RxTxCamera.lvclass"=w1148:refnum<class "RxTxCamera.lvclass">, "Application out"=w1144:refnum<class "Application.lvclass">)  [unwired: 8 in]
        n672 = call "Write Command String.vi"("error in (no error)"=w1147, "Command String"="STOP", "RxTxCamera in"=w1148) -> ("error out"=w1151:errorcluster, "RxTxCamera out"=w1150:refnum<class "RxTxCamera.lvclass">)  [unwired: 7 in]
        n673 = call "Enqeue message.vi"("error in (no error)"=w1151, "RxTx in"=w1150) -> ("error out"=w1146:errorcluster, "RxTx out"=w1145:refnum<class "RxTxCamera.lvclass">)  [unwired: 8 in]
        n674 = call "Write RxTxCamera.lvclass.vi"("error in (no error)"=w1146, "RxTxCamera.lvclass"=w1145, "Application in"=w1144) -> ("error out"=w1142:errorcluster, "Application out"=w1143:refnum<class "Application.lvclass">)  [unwired: 7 in]
      }
    }
    n675 = Wait (ms)(milliseconds to wait=u32 150) -> ()  [unwired: 1 out]
    "LED cal" <- "Calibration Fiber"
    "LED sky" <- "Sky Fiber"
  }
  n676 = call "Read CCDCamera.lvclass.vi"("error in (no error)"=w28, "Application in"=w27) -> ("error out"=w25:errorcluster, "CCDCamera.lvclass"=w26:refnum<class "CCDCamera.lvclass">)  [unwired: 7 in, 1 out]
  n677 = call "Shut Down.vi"("error in (no error)"=w25, "CCDCamera in"=w26) -> ("CCDCamera out"=w29:refnum<class "CCDCamera.lvclass">)  [unwired: 8 in, 1 out]
  n678 = stacked-sequence {
    tunnel: w29 -> [_]
    frame #0 {
      w1153 = u8 3 items=["0.6", "2.2", "3.6", "4.33"] ("Vertical Shift Speed")
      w1154 = u8 0 items=["1", "2", "4"] ("Pre-amplifier gain")
      w1155 = u8 1 items=["100 KHz at 16 bit", "1 MHz at 16 bit"] ("Readout Rate")
      w1174 = 512
      w1161 = cluster{dbl, dbl} {0.0, 0.0}
      w1177 = FALSE ("SIF")
      w1186 = u16 0 ("X :")
      w1188 = u16 0 items=["Cooler OFF", "Cooler ON"] ("Cooler ON/OFF")
      w1189 = FALSE ("BIAS")
      w1192 = u16 0 items=["TTL Low", "TTL High"] ("Shutter TTL")
      w1193 = u16 2 items=["Fully Auto", "OPEN", "CLOSED"] ("Shutter Mode")
      w1202 = u16 0 items=["Unsigned 16", "Unsigned 32", "Signed 16", "Signed 32", "Float"] ("FITS Format")
      w1203 = u16 0 items=["Internal", "External", "N/A", "N/A", "N/A", "N/A", "External Start", "External Exposure (bulb)", "N/A", "External FVB EM", "Software", "N/A", "External Charge Shifting"] ("Trigger")
      w1204 = u16 4 items=["Full Vertical Binning", "Multi-Track", "Random-Track", "Single-Track", "Image"] ("Read Mode")
      w1205 = u16 1 items=["RESERVED", "Single Scan", "Accumulate", "Kinetics", "Fast Kinetics", "Run Til Abort", "RESERVED", "RESERVED", "RESERVED", "RESERVED", "Time Delayed Integration"] ("Acquisition Mode")
      w1208 = u16 0 items=["Cooler OFF", "Cooler ON"] ("Cooler ON/OFF")
      w1214 = u32 13816530
      n679 = property on="Binning" class="XYGraph (strict)"() -> ("XScale.Maximum"=w1159:dbl)  [unwired: 2 in, 2 out]
      n680 = property on="Binning" class="XYGraph (strict)"() -> ("YScale.Maximum"=w1157:dbl)  [unwired: 2 in, 2 out]
      n681 = local write "Exposure Time (s)  2"(0.0 ("Exposure Time (s)  2")) -> ()
      n682 = local write "Temperature"(i16 20 ("CurrentlyTemp")) -> ()
      n683 = local write "Acquisition Mode"(w1205) -> ()
      n684 = local write "Read Mode"(w1204) -> ()
      n685 = local write "Exposure time"(0.0 ("Exposure time")) -> ()
      n686 = local write "# Exposure"(u32 1 ("# Exposure")) -> ()
      n687 = local write "Trigger"(w1203) -> ()
      n688 = local write "FITS Format"(w1202) -> ()
      n689 = local write "Vertical Shift Speed"(w1153) -> ()
      n690 = local write "Pre-amplifier gain"(w1154) -> ()
      n691 = local write "Vertical binning"(1 ("Vertical binning")) -> ()
      n692 = local write "Final Column"(1024 ("Final Column")) -> ()
      n693 = local write "Final Line"(1024 ("Final Line")) -> ()
      n694 = local write "Initial Line"(1 ("Initial Line")) -> ()
      n695 = local write "Horizontal binning"(1 ("Horizontal binning")) -> ()
      n696 = local write "Initial Column"(1 ("Initial Column")) -> ()
      n697 = local write "Time to close (ms)"(u16 50 ("Time to close (ms)")) -> ()
      n698 = local write "Time to open (ms)"(u16 50 ("Time to open (ms)")) -> ()
      n699 = local write "Shutter Mode"(w1193) -> ()
      n700 = local write "Shutter TTL"(w1192) -> ()
      n701 = local write "Readout Rate"(w1155) -> ()
      n702 = local write "Exposing"(FALSE ("Exposing")) -> ()
      n703 = local write "Exposições realizadas"(u8 0 ("Exposições realizadas")) -> ()
      n704 = local write "Sub Image"(T3."1024 x 1024" ("Sub Image")) -> ()
      n705 = Divide(x=w1157, y=2) -> (x/y=w1165:dbl)
      n706 = Divide(x=w1159, y=2) -> (x/y=w1166:dbl)
      n707 = Subtract(x=w1166, y=w1174) -> (x-y=w1163:dbl)
      n708 = Add(x=w1174, y=w1166) -> (x+y=w1164:dbl)
      n709 = Add(x=w1174, y=w1165) -> (x+y=w1162:dbl)
      n710 = Subtract(x=w1165, y=w1174) -> (x-y=w1160:dbl)
      n711 = Bundle(u32 1985280, u32 1985280) -> (w1217:cluster{u32, u32})  [unwired: 1 in]
      n712 = control-ref of="Initialization"() -> (w1216:refnum<vi>)
      n713 = Bundle(cluster=w1161, w1163, w1160) -> (w1172:cluster{dbl, dbl})
      n714 = Bundle(cluster=w1161, w1164, w1160) -> (w1171:cluster{dbl, dbl})
      n715 = Bundle(cluster=w1161, w1164, w1162) -> (w1170:cluster{dbl, dbl})
      n716 = Bundle(cluster=w1161, w1163, w1162) -> (w1169:cluster{dbl, dbl})
      n717 = Bundle(cluster=w1161, w1160, w1160) -> (w1168:cluster{dbl, dbl})
      n718 = Build Array(w1217) -> (w1220:cluster{u32, u32}[])
      n719 = property on="Property Node" class="Bool (strict)"(reference=w1216, "Colors [4]"=w1220) -> ()  [unwired: 1 in, 2 out]
      n720 = property on="Temperature" class="DigNum (strict)"("NumText.BG Color"=w1214) -> ()  [unwired: 2 in, 2 out]
      n721 = local write "Cooler ON/OFF"(w1188) -> ()
      n722 = property on="Temperature" class="DigNum (strict)"("NumText.BGColor"=w1214) -> ()  [unwired: 2 in, 2 out]
      n723 = local write "Cooler ON/OFF"(w1208) -> ()
      n724 = local write "Set temperature"(20.0 ("Set temperature")) -> ()
      n725 = local write "X :"(w1186) -> ()
      n726 = local write "Y :"(w1186) -> ()
      n727 = local write "Data:"(w1186) -> ()
      n728 = local write "BIAS"(w1189) -> ()
      n729 = local write "COMP"(w1189) -> ()
      n730 = local write "FLAT"(w1189) -> ()
      n731 = local write "Image Graph"(i32[][] [] ("Intensity Graph")) -> ()
      n732 = local write "Error Num"(u16 0 ("Error Num")) -> ()
      n733 = local write "Error string"("" ("Error string")) -> ()
      n734 = Build Array(w1172, w1171, w1170, w1169, w1168) -> (w1173:cluster{dbl, dbl}[])
      n735 = local write "Initialization"(FALSE ("Initialization")) -> ()
      n736 = local write "Error led"(FALSE ("Error led")) -> ()
      n737 = local write "% Acquired"(0.0 ("Exposure time")) -> ()
      n738 = local write "Binning"(w1173) -> ()
      n739 = local write "FITS"(TRUE ("SIF")) -> ()
      n740 = local write "SIF"(w1177) -> ()
      n741 = local write "TIFF"(w1177) -> ()
      n742 = property on="Tiff Position" class="DigNum (strict)"("DisabledEnum"=T17."Disabled and Grayed Out" ("Disabled")) -> ()  [unwired: 2 in, 2 out]
      n743 = property on="Tiff Type" class="Ring (strict)"("DisabledEnum"=T17."Disabled and Grayed Out" ("Disabled")) -> ()  [unwired: 2 in, 2 out]
      n744 = property on="FITS Format" class="Ring (strict)"("DisabledEnum"=T17."Enabled" ("Disabled")) -> ()  [unwired: 2 in, 2 out]
      n745 = property on="Initial Line" class="DigNum (strict)"("DisabledEnum"=T17."Disabled and Grayed Out" ("Disabled")) -> ()  [unwired: 2 in, 2 out]
      n746 = property on="Initial Column" class="DigNum (strict)"("DisabledEnum"=T17."Disabled and Grayed Out" ("Disabled")) -> ()  [unwired: 2 in, 2 out]
      n747 = property on="Final Line" class="DigNum (strict)"("DisabledEnum"=T17."Disabled and Grayed Out" ("Disabled")) -> ()  [unwired: 2 in, 2 out]
      n748 = property on="Final Column" class="DigNum (strict)"("DisabledEnum"=T17."Disabled and Grayed Out" ("Disabled")) -> ()  [unwired: 2 in, 2 out]
    }
  }
